vi "Main_without_temperature.vi"() -> ()   [LabVIEW 2023]
uses:
  TEC LabVIEW Control Software v0.14/Source/LV Source/[meerstetter engineering TE Cooling]/TypeDefs/meTEC_ID 2000_Input Selection.ctl
  TEC LabVIEW Control Software v0.14/Source/LV Source/[meerstetter engineering TE Cooling]/TypeDefs/meTEC_ID 50011_Object Target Temperature Source Selection.ctl
  TEC LabVIEW Control Software v0.14/Source/LV Source/[meerstetter engineering TE Cooling]/TypeDefs/meTEC_ID 50000_Live Enable.ctl
  TEC LabVIEW Control Software v0.14/Source/LV Source/[meerstetter engineering TE Cooling]/TypeDefs/meTEC_ID 1200_Temperature is Stable.ctl
  TEC LabVIEW Control Software v0.14/Source/LV Source/[meerstetter engineering TE Cooling]/TypeDefs/meTEC_ID 104_Device Status.ctl
  Application_class/Instruments.ctl
  AD2_MSO_SDK_class/MSOConfig.ctl
  AD2_MSO_SDK_class/AD2TriggerSources.ctl
  AD2_MSO_SDK_class/MSORangeCh.ctl
  Application_class/Control 1.ctl
  Hamamatsu_class/SubRegion.ctl
  Application_class/Application.lvclass
  Dummy_Mtec_class/Dummy_Mtec.lvclass
  C:/GIT/PowerScan/MTEC_Async_class/MTEC_Async.lvclass
  MTEC_Async_class/MTEC_Async.lvclass
  AD2andExtAWG_class/AD2andExtAWG.lvclass
  C:/GIT/PowerScan/InstrumentBase_class/AD2_SDK_class/InstrumentBase.lvclass
  <vilib>/Utility/error.llb/Error Cluster From Error Code.vi
  <vilib>/measure/matone.llb/Extract Single Tone Information 1 Chan.vi
  <vilib>/ErrorRing/Error Ring.xnode
  Hamamatsu_class/Hamamatsu.lvclass
  MTec_class/MTec.lvclass
  InstrumentBase_class/AD2_SDK_class/InstrumentBase.lvclass
  Experiment_class/Experiment.lvclass
  TDMSLogger_PowerScan_class/TDMSLogger_PowerScan.lvclass
  CetoniPump_class/CetoniPump.lvclass
  <vilib>/measure/NI_MAPro.lvlib
  AD2_MSO_SDK_class/AD2_MSO_SDK.lvclass
panel:
  in  "mem size":i32=100
  out "XY Graph":cluster{timestamp[], dbl[]}[](graph)=[{[timestamp(3810714974.4625654 s since 1904-01-01), timestamp(3810714974.6875706 s since 1904-01-01), timestamp(3810714974.9102407 s since 1904-01-01), timestamp(3810714975.132108 s since 1904-01-01), timestamp(3810714975.357173 s since 1904-01-01), timestamp(3810714975.581321 s since 1904-01-01), timestamp(3810714975.80342 s since 1904-01-01), timestamp(3810714976.0264726 s since 1904-01-01), timestamp(3810714976.250123 s since 1904-01-01), timestamp(3810714976.475124 s since 1904-01-01), timestamp(3810714976.6991234 s since 1904-01-01), timestamp(3810714976.9211745 s since 1904-01-01), timestamp(3810714977.1451674 s since 1904-01-01), timestamp(3810714977.368175 s since 1904-01-01), timestamp(3810714977.594176 s since 1904-01-01), timestamp(3810714977.816176 s since 1904-01-01), timestamp(3810714978.0411744 s since 1904-01-01), timestamp(3810714978.263168 s since 1904-01-01), timestamp(3810714978.488388 s since 1904-01-01), timestamp(3810714978.7113824 s since 1904-01-01), timestamp(3810714978.9333825 s since 1904-01-01), timestamp(3810714979.156552 s since 1904-01-01), timestamp(3810714979.380552 s since 1904-01-01), timestamp(3810714979.6040554 s since 1904-01-01), timestamp(3810714979.828112 s since 1904-01-01), timestamp(3810714980.051219 s since 1904-01-01), timestamp(3810714980.275273 s since 1904-01-01), timestamp(3810714980.499636 s since 1904-01-01), timestamp(3810714980.7226286 s since 1904-01-01), timestamp(3810714980.945965 s since 1904-01-01), timestamp(3810714981.170967 s since 1904-01-01), timestamp(3810714981.3933506 s since 1904-01-01), timestamp(3810714981.617357 s since 1904-01-01), timestamp(3810714981.840452 s since 1904-01-01), timestamp(3810714982.0654736 s since 1904-01-01), timestamp(3810714982.2894735 s since 1904-01-01), timestamp(3810714982.510492 s since 1904-01-01), timestamp(3810714982.734492 s since 1904-01-01), timestamp(3810714982.9584928 s since 1904-01-01), timestamp(3810714983.182848 s since 1904-01-01), timestamp(3810714983.4048495 s since 1904-01-01), timestamp(3810714983.6292033 s since 1904-01-01), timestamp(3810714983.8542337 s since 1904-01-01), timestamp(3810714984.077241 s since 1904-01-01), timestamp(3810714984.29924 s since 1904-01-01), timestamp(3810714984.52324 s since 1904-01-01), timestamp(3810714984.7462335 s since 1904-01-01), timestamp(3810714984.9702344 s since 1904-01-01), timestamp(3810714985.195372 s since 1904-01-01), timestamp(3810714985.417372 s since 1904-01-01), timestamp(3810714985.6413646 s since 1904-01-01), timestamp(3810714985.86677 s since 1904-01-01), timestamp(3810714986.0896926 s since 1904-01-01), timestamp(3810714986.311692 s since 1904-01-01), timestamp(3810714986.5356846 s since 1904-01-01), timestamp(3810714986.7598567 s since 1904-01-01), timestamp(3810714986.9828496 s since 1904-01-01), timestamp(3810714987.2071743 s since 1904-01-01), timestamp(3810714987.4291744 s since 1904-01-01), timestamp(3810714987.653329 s since 1904-01-01), timestamp(3810714987.8773217 s since 1904-01-01), timestamp(3810714988.1004457 s since 1904-01-01), timestamp(3810714988.325448 s since 1904-01-01), timestamp(3810714988.547662 s since 1904-01-01), timestamp(3810714988.7716546 s since 1904-01-01), timestamp(3810714988.994662 s since 1904-01-01), timestamp(3810714989.217661 s since 1904-01-01), timestamp(3810714989.443828 s since 1904-01-01), timestamp(3810714989.666828 s since 1904-01-01), timestamp(3810714989.890928 s since 1904-01-01), timestamp(3810714990.11292 s since 1904-01-01), timestamp(3810714990.335927 s since 1904-01-01), timestamp(3810714990.55996 s since 1904-01-01), timestamp(3810714990.7829666 s since 1904-01-01), timestamp(3810714991.006976 s since 1904-01-01), timestamp(3810714991.2310686 s since 1904-01-01), timestamp(3810714991.454176 s since 1904-01-01), timestamp(3810714991.679184 s since 1904-01-01), timestamp(3810714991.903184 s since 1904-01-01), timestamp(3810714992.125177 s since 1904-01-01), timestamp(3810714992.348177 s since 1904-01-01), timestamp(3810714992.572276 s since 1904-01-01), timestamp(3810714992.7962766 s since 1904-01-01), timestamp(3810714993.0195527 s since 1904-01-01), timestamp(3810714993.242547 s since 1904-01-01), timestamp(3810714993.4665465 s since 1904-01-01), timestamp(3810714993.6905394 s since 1904-01-01), timestamp(3810714993.913547 s since 1904-01-01), timestamp(3810714994.1385465 s since 1904-01-01), timestamp(3810714994.3625464 s since 1904-01-01), timestamp(3810714994.585547 s since 1904-01-01), timestamp(3810714994.80954 s since 1904-01-01), timestamp(3810714995.0335464 s since 1904-01-01), timestamp(3810714995.257552 s since 1904-01-01), timestamp(3810714995.4805474 s since 1904-01-01), timestamp(3810714995.7045465 s since 1904-01-01), timestamp(3810714995.925547 s since 1904-01-01), timestamp(3810714996.150547 s since 1904-01-01), timestamp(3810714996.374549 s since 1904-01-01), timestamp(3810714996.596541 s since 1904-01-01)], [22.902175903320312, 22.901992797851562, 22.903213500976562, 22.902908325195312, 22.903305053710938, 22.905197143554688, 22.906875610351562, 22.906539916992188, 22.906539916992188, 22.909378051757812, 22.910781860351562, 22.912826538085938, 22.915451049804688, 22.914047241210938, 22.917343139648438, 22.918472290039062, 22.918655395507812, 22.921981811523438, 22.920059204101562, 22.919723510742188, 22.918167114257812, 22.916549682617188, 22.915725708007812, 22.916458129882812, 22.916946411132812, 22.919662475585938, 22.916976928710938, 22.919906616210938, 22.921005249023438, 22.921249389648438, 22.922714233398438, 22.920883178710938, 22.924118041992188, 22.925735473632812, 22.928085327148438, 22.926986694335938, 22.929306030273438, 22.931716918945312, 22.930801391601562, 22.935470581054688, 22.936508178710938, 22.937179565429688, 22.939346313476562, 22.941116333007812, 22.940444946289062, 22.944534301757812, 22.943649291992188, 22.945999145507812, 22.944869995117188, 22.945846557617188, 22.945571899414062, 22.947494506835938, 22.948379516601562, 22.951004028320312, 22.948989868164062, 22.950271606445312, 22.950210571289062, 22.952072143554688, 22.951004028320312, 22.953475952148438, 22.954299926757812, 22.954116821289062, 22.953506469726562, 22.953598022460938, 22.954208374023438, 22.951828002929688, 22.953872680664062, 22.953018188476562, 22.953842163085938, 22.952865600585938, 22.955795288085938, 22.954513549804688, 22.955978393554688, 22.957351684570312, 22.954727172851562, 22.955886840820312, 22.955001831054688, 22.955825805664062, 22.954360961914062, 22.955032348632812, 22.957229614257812, 22.955490112304688, 22.958755493164062, 22.959518432617188, 22.959548950195312, 22.956710815429688, 22.959915161132812, 22.959487915039062, 22.959426879882812, 22.960617065429688, 22.960525512695312, 22.959243774414062, 22.960983276367188, 22.960647583007812, 22.962112426757812, 22.964004516601562, 22.964279174804688, 22.965377807617188, 22.964614868164062, 22.965621948242188]}, {[timestamp(3810714974.4625654 s since 1904-01-01), timestamp(3810714974.6875706 s since 1904-01-01), timestamp(3810714974.9102407 s since 1904-01-01), timestamp(3810714975.132108 s since 1904-01-01), timestamp(3810714975.357173 s since 1904-01-01), timestamp(3810714975.581321 s since 1904-01-01), timestamp(3810714975.80342 s since 1904-01-01), timestamp(3810714976.0264726 s since 1904-01-01), timestamp(3810714976.250123 s since 1904-01-01), timestamp(3810714976.475124 s since 1904-01-01), timestamp(3810714976.6991234 s since 1904-01-01), timestamp(3810714976.9211745 s since 1904-01-01), timestamp(3810714977.1451674 s since 1904-01-01), timestamp(3810714977.368175 s since 1904-01-01), timestamp(3810714977.594176 s since 1904-01-01), timestamp(3810714977.816176 s since 1904-01-01), timestamp(3810714978.0411744 s since 1904-01-01), timestamp(3810714978.263168 s since 1904-01-01), timestamp(3810714978.488388 s since 1904-01-01), timestamp(3810714978.7113824 s since 1904-01-01), timestamp(3810714978.9333825 s since 1904-01-01), timestamp(3810714979.156552 s since 1904-01-01), timestamp(3810714979.380552 s since 1904-01-01), timestamp(3810714979.6040554 s since 1904-01-01), timestamp(3810714979.828112 s since 1904-01-01), timestamp(3810714980.051219 s since 1904-01-01), timestamp(3810714980.275273 s since 1904-01-01), timestamp(3810714980.499636 s since 1904-01-01), timestamp(3810714980.7226286 s since 1904-01-01), timestamp(3810714980.945965 s since 1904-01-01), timestamp(3810714981.170967 s since 1904-01-01), timestamp(3810714981.3933506 s since 1904-01-01), timestamp(3810714981.617357 s since 1904-01-01), timestamp(3810714981.840452 s since 1904-01-01), timestamp(3810714982.0654736 s since 1904-01-01), timestamp(3810714982.2894735 s since 1904-01-01), timestamp(3810714982.510492 s since 1904-01-01), timestamp(3810714982.734492 s since 1904-01-01), timestamp(3810714982.9584928 s since 1904-01-01), timestamp(3810714983.182848 s since 1904-01-01), timestamp(3810714983.4048495 s since 1904-01-01), timestamp(3810714983.6292033 s since 1904-01-01), timestamp(3810714983.8542337 s since 1904-01-01), timestamp(3810714984.077241 s since 1904-01-01), timestamp(3810714984.29924 s since 1904-01-01), timestamp(3810714984.52324 s since 1904-01-01), timestamp(3810714984.7462335 s since 1904-01-01), timestamp(3810714984.9702344 s since 1904-01-01), timestamp(3810714985.195372 s since 1904-01-01), timestamp(3810714985.417372 s since 1904-01-01), timestamp(3810714985.6413646 s since 1904-01-01), timestamp(3810714985.86677 s since 1904-01-01), timestamp(3810714986.0896926 s since 1904-01-01), timestamp(3810714986.311692 s since 1904-01-01), timestamp(3810714986.5356846 s since 1904-01-01), timestamp(3810714986.7598567 s since 1904-01-01), timestamp(3810714986.9828496 s since 1904-01-01), timestamp(3810714987.2071743 s since 1904-01-01), timestamp(3810714987.4291744 s since 1904-01-01), timestamp(3810714987.653329 s since 1904-01-01), timestamp(3810714987.8773217 s since 1904-01-01), timestamp(3810714988.1004457 s since 1904-01-01), timestamp(3810714988.325448 s since 1904-01-01), timestamp(3810714988.547662 s since 1904-01-01), timestamp(3810714988.7716546 s since 1904-01-01), timestamp(3810714988.994662 s since 1904-01-01), timestamp(3810714989.217661 s since 1904-01-01), timestamp(3810714989.443828 s since 1904-01-01), timestamp(3810714989.666828 s since 1904-01-01), timestamp(3810714989.890928 s since 1904-01-01), timestamp(3810714990.11292 s since 1904-01-01), timestamp(3810714990.335927 s since 1904-01-01), timestamp(3810714990.55996 s since 1904-01-01), timestamp(3810714990.7829666 s since 1904-01-01), timestamp(3810714991.006976 s since 1904-01-01), timestamp(3810714991.2310686 s since 1904-01-01), timestamp(3810714991.454176 s since 1904-01-01), timestamp(3810714991.679184 s since 1904-01-01), timestamp(3810714991.903184 s since 1904-01-01), timestamp(3810714992.125177 s since 1904-01-01), timestamp(3810714992.348177 s since 1904-01-01), timestamp(3810714992.572276 s since 1904-01-01), timestamp(3810714992.7962766 s since 1904-01-01), timestamp(3810714993.0195527 s since 1904-01-01), timestamp(3810714993.242547 s since 1904-01-01), timestamp(3810714993.4665465 s since 1904-01-01), timestamp(3810714993.6905394 s since 1904-01-01), timestamp(3810714993.913547 s since 1904-01-01), timestamp(3810714994.1385465 s since 1904-01-01), timestamp(3810714994.3625464 s since 1904-01-01), timestamp(3810714994.585547 s since 1904-01-01), timestamp(3810714994.80954 s since 1904-01-01), timestamp(3810714995.0335464 s since 1904-01-01), timestamp(3810714995.257552 s since 1904-01-01), timestamp(3810714995.4805474 s since 1904-01-01), timestamp(3810714995.7045465 s since 1904-01-01), timestamp(3810714995.925547 s since 1904-01-01), timestamp(3810714996.150547 s since 1904-01-01), timestamp(3810714996.374549 s since 1904-01-01), timestamp(3810714996.596541 s since 1904-01-01)], [23.093063354492188, 23.094924926757812, 23.094497680664062, 23.097518920898438, 23.095504760742188, 23.094528198242188, 23.098098754882812, 23.099533081054688, 23.102035522460938, 23.100082397460938, 23.105026245117188, 23.107894897460938, 23.107254028320312, 23.108169555664062, 23.112472534179688, 23.110580444335938, 23.116165161132812, 23.113418579101562, 23.113418579101562, 23.112075805664062, 23.110916137695312, 23.108871459960938, 23.107559204101562, 23.110641479492188, 23.111648559570312, 23.111618041992188, 23.113174438476562, 23.115737915039062, 23.115188598632812, 23.116897583007812, 23.113906860351562, 23.116683959960938, 23.119857788085938, 23.119705200195312, 23.120559692382812, 23.123886108398438, 23.123031616210938, 23.122512817382812, 23.124221801757812, 23.128158569335938, 23.127243041992188, 23.129959106445312, 23.131637573242188, 23.131820678710938, 23.133285522460938, 23.136337280273438, 23.136276245117188, 23.136917114257812, 23.138320922851562, 23.137313842773438, 23.141921997070312, 23.142196655273438, 23.142440795898438, 23.143112182617188, 23.145858764648438, 23.144485473632812, 23.147598266601562, 23.147171020507812, 23.149276733398438, 23.149337768554688, 23.149276733398438, 23.152023315429688, 23.155258178710938, 23.155410766601562, 23.153366088867188, 23.155471801757812, 23.154800415039062, 23.155899047851562, 23.157669067382812, 23.159255981445312, 23.157211303710938, 23.157821655273438, 23.160781860351562, 23.162673950195312, 23.161300659179688, 23.164657592773438, 23.164108276367188, 23.163711547851562, 23.162490844726562, 23.165390014648438, 23.165481567382812, 23.165939331054688, 23.165573120117188, 23.169692993164062, 23.168869018554688, 23.167984008789062, 23.168258666992188, 23.168411254882812, 23.168258666992188, 23.168899536132812, 23.170425415039062, 23.170089721679688, 23.171829223632812, 23.173904418945312, 23.172744750976562, 23.175460815429688, 23.173141479492188, 23.174606323242188, 23.174728393554688, 23.175674438476562]}, {[timestamp(3810714974.4625654 s since 1904-01-01), timestamp(3810714974.6875706 s since 1904-01-01), timestamp(3810714974.9102407 s since 1904-01-01), timestamp(3810714975.132108 s since 1904-01-01), timestamp(3810714975.357173 s since 1904-01-01), timestamp(3810714975.581321 s since 1904-01-01), timestamp(3810714975.80342 s since 1904-01-01), timestamp(3810714976.0264726 s since 1904-01-01), timestamp(3810714976.250123 s since 1904-01-01), timestamp(3810714976.475124 s since 1904-01-01), timestamp(3810714976.6991234 s since 1904-01-01), timestamp(3810714976.9211745 s since 1904-01-01), timestamp(3810714977.1451674 s since 1904-01-01), timestamp(3810714977.368175 s since 1904-01-01), timestamp(3810714977.594176 s since 1904-01-01), timestamp(3810714977.816176 s since 1904-01-01), timestamp(3810714978.0411744 s since 1904-01-01), timestamp(3810714978.263168 s since 1904-01-01), timestamp(3810714978.488388 s since 1904-01-01), timestamp(3810714978.7113824 s since 1904-01-01), timestamp(3810714978.9333825 s since 1904-01-01), timestamp(3810714979.156552 s since 1904-01-01), timestamp(3810714979.380552 s since 1904-01-01), timestamp(3810714979.6040554 s since 1904-01-01), timestamp(3810714979.828112 s since 1904-01-01), timestamp(3810714980.051219 s since 1904-01-01), timestamp(3810714980.275273 s since 1904-01-01), timestamp(3810714980.499636 s since 1904-01-01), timestamp(3810714980.7226286 s since 1904-01-01), timestamp(3810714980.945965 s since 1904-01-01), timestamp(3810714981.170967 s since 1904-01-01), timestamp(3810714981.3933506 s since 1904-01-01), timestamp(3810714981.617357 s since 1904-01-01), timestamp(3810714981.840452 s since 1904-01-01), timestamp(3810714982.0654736 s since 1904-01-01), timestamp(3810714982.2894735 s since 1904-01-01), timestamp(3810714982.510492 s since 1904-01-01), timestamp(3810714982.734492 s since 1904-01-01), timestamp(3810714982.9584928 s since 1904-01-01), timestamp(3810714983.182848 s since 1904-01-01), timestamp(3810714983.4048495 s since 1904-01-01), timestamp(3810714983.6292033 s since 1904-01-01), timestamp(3810714983.8542337 s since 1904-01-01), timestamp(3810714984.077241 s since 1904-01-01), timestamp(3810714984.29924 s since 1904-01-01), timestamp(3810714984.52324 s since 1904-01-01), timestamp(3810714984.7462335 s since 1904-01-01), timestamp(3810714984.9702344 s since 1904-01-01), timestamp(3810714985.195372 s since 1904-01-01), timestamp(3810714985.417372 s since 1904-01-01), timestamp(3810714985.6413646 s since 1904-01-01), timestamp(3810714985.86677 s since 1904-01-01), timestamp(3810714986.0896926 s since 1904-01-01), timestamp(3810714986.311692 s since 1904-01-01), timestamp(3810714986.5356846 s since 1904-01-01), timestamp(3810714986.7598567 s since 1904-01-01), timestamp(3810714986.9828496 s since 1904-01-01), timestamp(3810714987.2071743 s since 1904-01-01), timestamp(3810714987.4291744 s since 1904-01-01), timestamp(3810714987.653329 s since 1904-01-01), timestamp(3810714987.8773217 s since 1904-01-01), timestamp(3810714988.1004457 s since 1904-01-01), timestamp(3810714988.325448 s since 1904-01-01), timestamp(3810714988.547662 s since 1904-01-01), timestamp(3810714988.7716546 s since 1904-01-01), timestamp(3810714988.994662 s since 1904-01-01), timestamp(3810714989.217661 s since 1904-01-01), timestamp(3810714989.443828 s since 1904-01-01), timestamp(3810714989.666828 s since 1904-01-01), timestamp(3810714989.890928 s since 1904-01-01), timestamp(3810714990.11292 s since 1904-01-01), timestamp(3810714990.335927 s since 1904-01-01), timestamp(3810714990.55996 s since 1904-01-01), timestamp(3810714990.7829666 s since 1904-01-01), timestamp(3810714991.006976 s since 1904-01-01), timestamp(3810714991.2310686 s since 1904-01-01), timestamp(3810714991.454176 s since 1904-01-01), timestamp(3810714991.679184 s since 1904-01-01), timestamp(3810714991.903184 s since 1904-01-01), timestamp(3810714992.125177 s since 1904-01-01), timestamp(3810714992.348177 s since 1904-01-01), timestamp(3810714992.572276 s since 1904-01-01), timestamp(3810714992.7962766 s since 1904-01-01), timestamp(3810714993.0195527 s since 1904-01-01), timestamp(3810714993.242547 s since 1904-01-01), timestamp(3810714993.4665465 s since 1904-01-01), timestamp(3810714993.6905394 s since 1904-01-01), timestamp(3810714993.913547 s since 1904-01-01), timestamp(3810714994.1385465 s since 1904-01-01), timestamp(3810714994.3625464 s since 1904-01-01), timestamp(3810714994.585547 s since 1904-01-01), timestamp(3810714994.80954 s since 1904-01-01), timestamp(3810714995.0335464 s since 1904-01-01), timestamp(3810714995.257552 s since 1904-01-01), timestamp(3810714995.4805474 s since 1904-01-01), timestamp(3810714995.7045465 s since 1904-01-01), timestamp(3810714995.925547 s since 1904-01-01), timestamp(3810714996.150547 s since 1904-01-01), timestamp(3810714996.374549 s since 1904-01-01), timestamp(3810714996.596541 s since 1904-01-01)], [0.0, 0.0, 0.0, 0.0, 0.0, 0.0, 0.0, 0.0, 0.0, 0.0, 0.0, 0.0, 0.0, 0.0, 0.0, 0.0, 0.0, 0.0, 0.0, 0.0, 0.0, 0.0, 0.0, 0.0, 0.0, 0.0, 0.0, 0.0, 0.0, 0.0, 0.0, 0.0, 0.0, 0.0, 0.0, 0.0, 0.0, 0.0, 0.0, 0.0, 0.0, 0.0, 0.0, 0.0, 0.0, 0.0, 0.0, 0.0, 0.0, 0.0, 0.0, 0.0, 0.0, 0.0, 0.0, 0.0, 0.0, 0.0, 0.0, 0.0, 0.0, 0.0, 0.0, 0.0, 0.0, 0.0, 0.0, 0.0, 0.0, 0.0, 0.0, 0.0, 0.0, 0.0, 0.0, 0.0, 0.0, 0.0, 0.0, 0.0, 0.0, 0.0, 0.0, 0.0, 0.0, 0.0, 0.0, 0.0, 0.0, 0.0, 0.0, 0.0, 0.0, 0.0, 0.0, 0.0, 0.0, 0.0, 0.0, 0.0]}]
  in  "Chart Length":enum16{"60 s", "10 minutes", "1 h"}(ring)=enum."10 minutes"
  out "Waveform Chart":waveform(dbl)[](graph)=[{"t0"=timestamp(3810714996.596541 s since 1904-01-01), "dt"=1.0, "Y"=[22.965621948242188]}, {"t0"=timestamp(3810714996.596541 s since 1904-01-01), "dt"=1.0, "Y"=[23.175674438476562]}]
  in  "Read MSO":bool
  out "error out":errorcluster
  out "Status":string="Exiting.."
  in  "AutoScaleCh1":bool=TRUE caption="AutoScale timebase to ChA"
  out "V/Hz/Deg":dbl[](array[numeric])=[256495.2123849432, 0.012104949851784449, 127.31074154871095, 4268838.632377055, 0.0003381910830981614, 134.9693104826537]
  out "Data":string[](array[string])=["Ch1Freq", "Ch1Amp", "Ch1Phase", "Ch2Freq", "Ch2Amp", "Ch2Phase"]
  out "MSO Data WaveForms 2":waveform(dbl)[](graph)=[{"t0"=timestamp(0 s since 1904-01-01), "dt"=1e-08, "Y"=array[8192 elements]}, {"t0"=timestamp(0 s since 1904-01-01), "dt"=1e-08, "Y"=array[8192 elements]}]
  in  "ABORT":bool
  in  "Tab Control":T1(tab)=enum."Cetoni"
  in  "Use Cetoni?":bool=TRUE
  in  "Use Hamamatsu":bool=TRUE
  in  "Use MeTEC?":bool=TRUE
  in  "AWG VISA resource name":refnum<visa-resource-name>="USB0::0x0699::0x0347::C037907::INSTR"
  in  "System Configuration":T2
  in  "Initialize System":bool
  in  "Use Instruments?":bool=TRUE
  in  "Device Configuration Path":string="C:\\Users\\Public\\Documents\\QmixElements\\Projects\\default_project\\Configurations\\double"
  in  "Turn Off WFG During Refill":bool
  in  "index":i32
  in  "refill below level(uL)":dbl=1000.0
  in  "Refill":bool
  in  "Conditional Refill":bool
  in  "Empty":bool
  in  "Stop pumps":bool
  in  "SyringeSettings":T3={"Maximum Piston Stroke (mm)"=66.0, "Inner Diameter (mm)"=14.5}
  in  "Configure Syringe":bool
  in  "ValveControl":cluster{"index":i32, "Valve Position":bool}
  in  "Go to Level":bool
  in  "GoToLevelSettings":T4={"index"=0, "Level(uL)"=0.0, "Flow"=250.0}
  in  "Monitor Pump":bool
  out "Array":T5(array[cluster])=[{"Pump Name"="neMESYS_Low_Pressure_1_Pump", "Actual Flow Rate"=249.9994261659258, "Fill Level"=9609.141943854513, "Is pumping"=TRUE}, {"Pump Name"="neMESYS_Low_Pressure_2_Pump", "Actual Flow Rate"=0.0, "Fill Level"=0.0, "Is pumping"=FALSE}]
  in  "ReferenceMove":bool
  in  "refill and \nempty rate(uL/min)":dbl=12000.0
  in  "Wait After Conditional Refill (s)":dbl=50.0
  out "Cluster":T8={"meTEC_CH2_Temperature Stability"=0, "meTEC_CH2_Act. Output Current [A]"=0.009997940622270107, "meTEC_CH2_Act. Output Voltage [V]"=0.004072710871696472, "meTEC_CH2_Object Temperature [°C]"=23.175674438476562, "meTEC_CH2_Sink Temperature [°C]"=25.0, "meTEC_CH1_Error Parameter"=0, "meTEC_CH1_Error Instance"=0, "meTEC_CH1_Error No."=0, "meTEC_CH1_Device Status"=1, "meTEC_CH1_Temperature Stability"=0, "meTEC_CH1_Act. Output Current [A]"=0.010120010934770107, "meTEC_CH1_Act. Output Voltage [V]"=0.009891997091472149, "meTEC_CH1_Object Temperature [°C]"=22.965621948242188, "meTEC_CH1_Sink Temperature [°C]"=25.0} {"meTEC_CH1_Sink Temperature [°C]" format="%.3f"; "meTEC_CH1_Object Temperature [°C]" format="%.3f"; "meTEC_CH1_Act. Output Voltage [V]" format="%.3f"; "meTEC_CH1_Act. Output Current [A]" format="%.3f"; "meTEC_CH1_Temperature Stability" items=["Temperature regulation is not active", "Is not stable", "Is stable"]; "meTEC_CH1_Device Status" items=["Initializing", "Ready", "Run", "Error", "Bootloader", "Reset in Progress"]; "meTEC_CH2_Sink Temperature [°C]" format="%.3f"; "meTEC_CH2_Object Temperature [°C]" format="%.3f"; "meTEC_CH2_Act. Output Voltage [V]" format="%.3f"; "meTEC_CH2_Act. Output Current [A]" format="%.3f"; "meTEC_CH2_Temperature Stability" items=["Temperature regulation is not active", "Is not stable", "Is stable"]}
  in  "Config Data":T12={"meTEC_CH1_Input Selection (ID 2000)"=2, "meTEC_CH2_Input Selection (ID 2000)"=2, "meTEC_CH1_Object Target Temp. Source Selection (ID 50011)"=0, "meTEC_CH2_Object Target Temp. Source Selection (ID 50011)"=0, "meTEC_CH1_Live Enable (ID 50000)"=0, "meTEC_CH2_Live Enable (ID 50000)"=0, "meTEC_CH1_Object Target Temperature (ID 3000 / 50012) [°C]"=23.0, "meTEC_CH2_Object Target Temperature (ID 3000 / 50012) [°C]"=23.0, "meTEC_CH1_Live Set Current (ID 50001) [A]"=0.0, "meTEC_CH2_Live Set Current (ID 50001) [A]"=0.0, "meTEC_CH1_Live Set Voltage (ID 50002) [V]"=0.0, "meTEC_CH2_Live Set Voltage (ID 50002) [V]"=0.0} {"meTEC_CH2_Live Set Voltage (ID 50002) [V]" format="%#.3f"; "meTEC_CH1_Live Set Voltage (ID 50002) [V]" format="%#.3f"; "meTEC_CH2_Live Set Current (ID 50001) [A]" format="%#.3f"; "meTEC_CH1_Live Set Current (ID 50001) [A]" format="%#.3f"; "meTEC_CH2_Object Target Temperature (ID 3000 / 50012) [°C]" format="%#.3f"; "meTEC_CH1_Object Target Temperature (ID 3000 / 50012) [°C]" format="%#.3f"; "meTEC_CH2_Live Enable (ID 50000)" items=["Disabled (Reset State)", "Enabled"]; "meTEC_CH1_Live Enable (ID 50000)" items=["Disabled (Reset State)", "Enabled"]; "meTEC_CH2_Object Target Temp. Source Selection (ID 50011)" items=["Parameter ID 3000 (Reset State)", "Parameter ID 50012"]; "meTEC_CH1_Object Target Temp. Source Selection (ID 50011)" items=["Parameter ID 3000 (Reset State)", "Parameter ID 50012"]; "meTEC_CH2_Input Selection (ID 2000)" items=["Static Current / Voltage", "Live Current / Voltage", "Temperature Controller"]; "meTEC_CH1_Input Selection (ID 2000)" items=["Static Current / Voltage", "Live Current / Voltage", "Temperature Controller"]}
  in  "Configure TEC":bool
  in  "Monitor":bool=TRUE
  in  "ResetMtec":bool
  in  "Metec Flush Memory":bool
  in  "OutputEnable":T13
  in  "Config WFG":bool
  in  "Freq Ch1&2":T14
  in  "Configdatastd":T15={"ConfigDataCh1"={"Frequency Hz (1000 Hz)"=1000.0, "Waveform Function (0: Sine)"=0, "Amplitude (1 Vpp)"=1.0, "DC Offset (0.00 V)"=0.0, "Phase Level (-1)"=0.0, "Phase Unit (0: Radian)"=0}, "ConfigDataCh2"={"Frequency Hz (1000 Hz)"=1000.0, "Waveform Function (0: Sine)"=0, "Amplitude (1 Vpp)"=1.0, "DC Offset (0.00 V)"=0.0, "Phase Level (-1)"=0.0, "Phase Unit (0: Radian)"=0}} {"ConfigDataCh1"."Frequency Hz (1000 Hz)" min=0.0 max=100000000.0}
  in  "CurrentProbeScaling(V/A)":dbl=5.0
  in  "PwrScanSettings":T16={"FreqStart(Hz)"=1800000.0, "Increment(Hz)"=1000.0, "Steps"=100}
  out "Power Graph":T17=[{"PwrFreq"=[1800000.0, 1801000.0, 1802000.0, 1803000.0, 1804000.0, 1805000.0, 1806000.0, 1807000.0, 1808000.0, 1809000.0, 1810000.0, 1811000.0, 1812000.0, 1813000.0, 1814000.0, 1815000.0, 1816000.0, 1817000.0, 1818000.0, 1819000.0, 1820000.0, 1821000.0, 1822000.0, 1823000.0, 1824000.0, 1825000.0, 1826000.0, 1827000.0, 1828000.0, 1829000.0, 1830000.0, 1831000.0, 1832000.0, 1833000.0, 1834000.0, 1835000.0, 1836000.0, 1837000.0, 1838000.0, 1839000.0, 1840000.0, 1841000.0, 1842000.0, 1843000.0, 1844000.0, 1845000.0, 1846000.0, 1847000.0, 1848000.0, 1849000.0, 1850000.0, 1851000.0, 1852000.0, 1853000.0, 1854000.0, 1855000.0, 1856000.0, 1857000.0, 1858000.0, 1859000.0, 1860000.0, 1861000.0, 1862000.0, 1863000.0, 1864000.0, 1865000.0, 1866000.0, 1867000.0, 1868000.0, 1869000.0, 1870000.0, 1871000.0, 1872000.0, 1873000.0, 1874000.0, 1875000.0, 1876000.0, 1877000.0, 1878000.0, 1879000.0, 1880000.0, 1881000.0, 1882000.0, 1883000.0, 1884000.0, 1885000.0, 1886000.0, 1887000.0, 1888000.0, 1889000.0, 1890000.0, 1891000.0, 1892000.0, 1893000.0, 1894000.0, 1895000.0, 1896000.0, 1897000.0, 1898000.0, 1899000.0], "PwrMeasured"=[0.03743018699905172, 0.03868842711054406, 0.039939450983681936, 0.041186940846945984, 0.042492363236693975, 0.04404846555067622, 0.04602835102242353, 0.04843888820937301, 0.05119026075250401, 0.054137745072059686, 0.05681989848669318, 0.05866977349663312, 0.05974650294953525, 0.06005376515825572, 0.05994285605916934, 0.05965859181003201, 0.05940789816848652, 0.05911436810870655, 0.05887115083576992, 0.058285278937152116, 0.05733209401753114, 0.05612065814579392, 0.05491201122450486, 0.054246204884069796, 0.05413387963390649, 0.0544784492868222, 0.055223443274043806, 0.05584761484864832, 0.05593777472478643, 0.055604310692913786, 0.05518644597062401, 0.054618464862787694, 0.054214223715299915, 0.05394256784700533, 0.0538322569007853, 0.05378224385812821, 0.053684397213232725, 0.053570515853526054, 0.05367988225271155, 0.05367731285637497, 0.05328103475935342, 0.05261733484260826, 0.05172095371283941, 0.050922021343682664, 0.05021598202266246, 0.049693559571941236, 0.04964157824916153, 0.049770317527984026, 0.04982229343352004, 0.0491940448801376, 0.048088239496034246, 0.0465169483544214, 0.0449815088404273, 0.04339710247015175, 0.04200318845517933, 0.04079371088999795, 0.03986802195324547, 0.038792483453571246, 0.03777766173772913, 0.03677527534117768, 0.0359760414327305, 0.03518671210489007, 0.03475002270949958, 0.03471532342952112, 0.03517735874853088, 0.03613562839997322, 0.0377065106935801, 0.0398207089338458, 0.04192610453201364, 0.04433368155489899, 0.04724045693183674, 0.05041187326865423, 0.05357414254285915, 0.056935687754456586, 0.06034831631771629, 0.06370638524387114, 0.06689701401467622, 0.06907501466358135, 0.07011171729016413, 0.06928919978057443, 0.06697831206028507, 0.06356111518422408, 0.059707919276213384, 0.055820271940164715, 0.05201579594450088, 0.048220123240964884, 0.044549547433591366, 0.04117661978432694, 0.038128405762736364, 0.03561051707739825, 0.03331342696116638, 0.03141526136270806, 0.029497507637866037, 0.02786984120696333, 0.0266553633197663, 0.025619681037449903, 0.024768741920820493, 0.024028995090048973, 0.023324807778494015, 0.022671870223729386]}, {"PwrFreq"=[], "PwrMeasured"=[]}, {"PwrFreq"=[], "PwrMeasured"=[]}]
  in  "AdjustPower":bool
  in  "DesiredPower(W)":dbl=0.001 min=0.001
  out "min Power":dbl=0.022671870223729386
  out "max Power":dbl=0.07011171729016413
  out "Measured Power":dbl=0.014358194668451557
  in  "MeasurePower":bool
  out "AmplitudeOk":bool=TRUE
  in  "Run Power Scan":bool
  out "phase (deg)":dbl=82.9743375382008
  out "impedance (ohm)":dbl=0.07240014859741192
  in  "Config":T18={"Timing"={"Enable"=TRUE, "Samples In"=8000.0, "Sample Rate"=100000000.0, "Mode"=enum."Single Sample"}, "Trigger"={"Hysteresis"=0.0, "Trigger Level"=0.0, "Trigger Condition"=0, "Trigger Type"=0, "Trigger Channel"=0, "secTimeout"=0.5, "TrigrSrc"=enum."trigsrcDetectorAnalogIn"}, "Range Ch1"={"idxChannel"=0, "voltOffset"=0.0, "VoltsRange"=50}, "Range Ch 2"={"idxChannel"=1, "voltOffset"=0.0, "VoltsRange"=5}} {"Range Ch 2"."VoltsRange" items=["High 50V"=50, "Low5V"=5]; "Range Ch1"."VoltsRange" items=["High 50V"=50, "Low5V"=5]; "Trigger"."Trigger Channel" items=["Channel 1"=0, "Channel 2"=1, "Both"=-1]; "Trigger"."Trigger Type" items=["Edge", "Pulse", "Transition"]; "Trigger"."Trigger Condition" items=["Rising", "Falling"]}
  in  "Configure MSO":bool
  in  "AutoRange MSO (Volt)":bool
  in  "Center ROI":bool=TRUE
  in  "Image":bool
  in  "Image Continous":bool
  in  "ExposureTime(ms)":dbl=5.0
  in  "ROI":T21={"Horizontal Offset"=0, "Vertical Offset"=652, "Horizontal Size"=2304, "Vertical Size"=1000} {"Vertical Size" min=4 max=1652 step=4; "Horizontal Size" min=4 max=2304 step=4; "Vertical Offset" min=0 max=1304 step=4; "Horizontal Offset" min=0 max=0 step=4}
  in  "Configure":bool
  in  "Fill List":bool
  in  "Number of Frequencies":dbl=101.0
  in  "Freq Increment":dbl=1000.0
  in  "Freq Start":dbl=1800000.0
  in  "Start Experiment":bool
  in  "Number of Images (#)":i32=10
  in  "wait time(s)":dbl
  in  "List of Powers to run(W)":dbl[](array[numeric])=[0.01, 0.02] min=0.001
  in  "List of Frequencies (Hz)":dbl[](array[numeric])=[1800000.0, 1801000.0, 1802000.0, 1803000.0, 1804000.0, 1805000.0, 1806000.0, 1807000.0, 1808000.0, 1809000.0, 1810000.0, 1811000.0, 1812000.0, 1813000.0, 1814000.0, 1815000.0, 1816000.0, 1817000.0, 1818000.0, 1819000.0, 1820000.0, 1821000.0, 1822000.0, 1823000.0, 1824000.0, 1825000.0, 1826000.0, 1827000.0, 1828000.0, 1829000.0, 1830000.0, 1831000.0, 1832000.0, 1833000.0, 1834000.0, 1835000.0, 1836000.0, 1837000.0, 1838000.0, 1839000.0, 1840000.0, 1841000.0, 1842000.0, 1843000.0, 1844000.0, 1845000.0, 1846000.0, 1847000.0, 1848000.0, 1849000.0, 1850000.0, 1851000.0, 1852000.0, 1853000.0, 1854000.0, 1855000.0, 1856000.0, 1857000.0, 1858000.0, 1859000.0, 1860000.0, 1861000.0, 1862000.0, 1863000.0, 1864000.0, 1865000.0, 1866000.0, 1867000.0, 1868000.0, 1869000.0, 1870000.0, 1871000.0, 1872000.0, 1873000.0, 1874000.0, 1875000.0, 1876000.0, 1877000.0, 1878000.0, 1879000.0, 1880000.0, 1881000.0, 1882000.0, 1883000.0, 1884000.0, 1885000.0, 1886000.0, 1887000.0, 1888000.0, 1889000.0, 1890000.0, 1891000.0, 1892000.0, 1893000.0, 1894000.0, 1895000.0, 1896000.0, 1897000.0, 1898000.0, 1899000.0, 1900000.0] min=0.001
  out "Progress (100%)":dbl=100.0
  in  "List of Flow Rates (ul/min)":dbl[](array[numeric])=[250.0]
  out "# elements in queue":i32=3256
  in  "Repeat Adjust Power and Wait N Times (#)":i32=1 min=1
  in  "wait after adjust power (s)":dbl
  in  "wait after changing flow rate(s)":dbl
  in  "AutoRange MSO":bool
  in  "Exit":bool
  # "All Power Levels"
  # "All Frequencies"
  # "All Flow Rates"
  # "Conditional Refill\nSet Flow\nChange Frequency\nEnable Function Generator\nAdjust Power\nWait (Adjust Power)\nWait\nSave Data (N times)\nDisable Function Generator\nWait\nSave Data"
  # "Measured Waveform"
  # "Index of the pump you are controlling"
  # "This one goes to 11!"
  # "Refills if syringe\nis below level"
  # "(sets it back to its previous state after)"
  # "Volt on ch1 and Current Probe ch2"
  # "(also measures impedance)"
  # "All Power Levels"
  # "All Frequencies"
  # "All Flow Rates"
  # "Conditional Refill\nSet Flow\nWait (flow)\nChange Frequency\nEnable Function Generator\nAdjust Power\nWait (Adjust Power)\nWait\nSave Data (N times)\nDisable Function Generator\nWait\nSave Data"
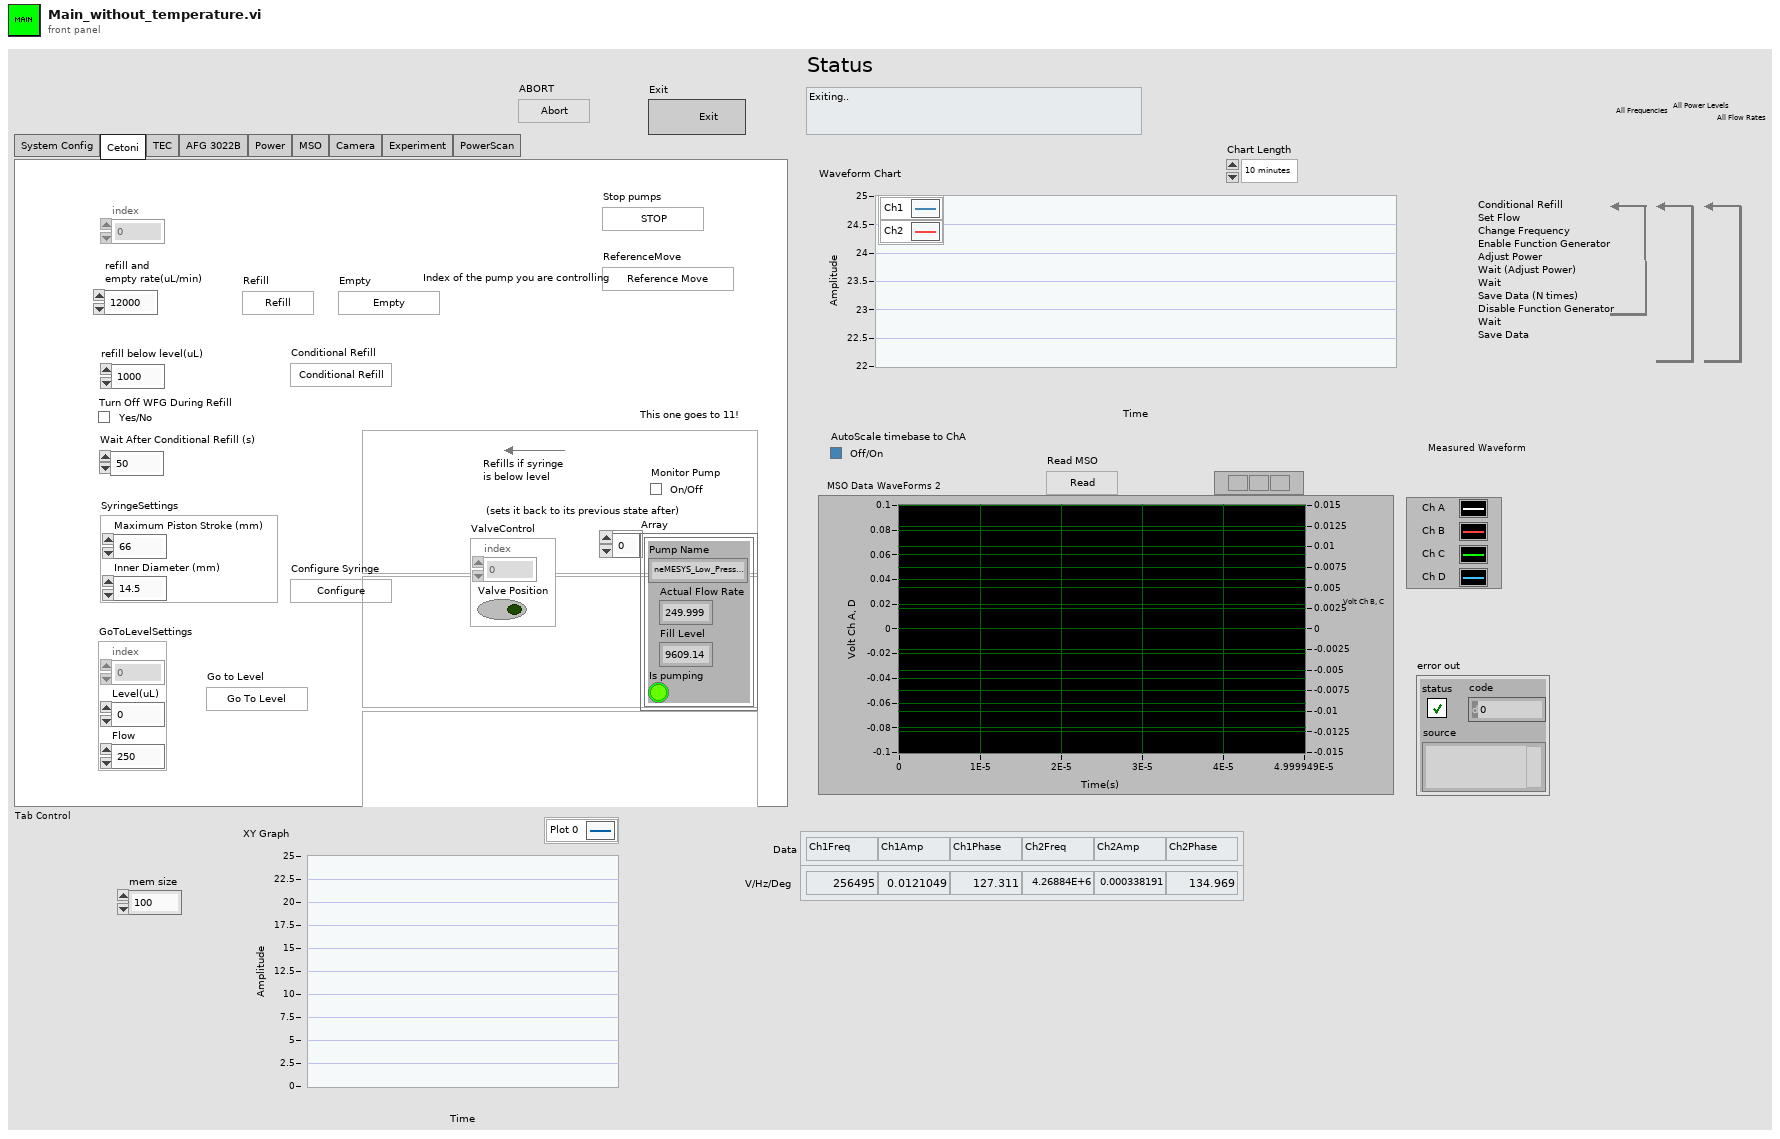
[diagram p1: front panel]
types:
  T1 = enum32{"System Config", "Cetoni", "TEC", "AFG 3022B", "Power", "MSO", "Camera", "Experiment", "PowerScan"}
  T2 = typedef "Application.lvclass/Instruments.ctl" = enum16{"AD2 and AFG3022"}
  T3 = cluster{"Maximum Piston Stroke (mm)":dbl, "Inner Diameter (mm)":dbl}
  T4 = cluster{"index":i32, "Level(uL)":dbl, "Flow":dbl}
  T5 = cluster{"Pump Name":string, "Actual Flow Rate":dbl, "Fill Level":dbl, "Is pumping":bool}[]
  T6 = typedef "meTEC_ID 1200_Temperature is Stable.ctl" = i32
  T7 = typedef "meTEC_ID 104_Device Status.ctl" = i32
  T8 = cluster{"meTEC_CH2_Temperature Stability":T6, "meTEC_CH2_Act. Output Current [A]":dbl, "meTEC_CH2_Act. Output Voltage [V]":dbl, "meTEC_CH2_Object Temperature [°C]":dbl, "meTEC_CH2_Sink Temperature [°C]":dbl, "meTEC_CH1_Error Parameter":i32, "meTEC_CH1_Error Instance":i32, "meTEC_CH1_Error No.":i32, "meTEC_CH1_Device Status":T7, "meTEC_CH1_Temperature Stability":T6, "meTEC_CH1_Act. Output Current [A]":dbl, "meTEC_CH1_Act. Output Voltage [V]":dbl, "meTEC_CH1_Object Temperature [°C]":dbl, "meTEC_CH1_Sink Temperature [°C]":dbl}
  T9 = typedef "meTEC_ID 2000_Input Selection.ctl" = i32
  T10 = typedef "meTEC_ID 50011_Object Target Temperature Source Selection.ctl" = i32
  T11 = typedef "meTEC_ID 50000_Live Enable.ctl" = i32
  T12 = cluster{"meTEC_CH1_Input Selection (ID 2000)":T9, "meTEC_CH2_Input Selection (ID 2000)":T9, "meTEC_CH1_Object Target Temp. Source Selection (ID 50011)":T10, "meTEC_CH2_Object Target Temp. Source Selection (ID 50011)":T10, "meTEC_CH1_Live Enable (ID 50000)":T11, "meTEC_CH2_Live Enable (ID 50000)":T11, "meTEC_CH1_Object Target Temperature (ID 3000 / 50012) [°C]":dbl, "meTEC_CH2_Object Target Temperature (ID 3000 / 50012) [°C]":dbl, "meTEC_CH1_Live Set Current (ID 50001) [A]":dbl, "meTEC_CH2_Live Set Current (ID 50001) [A]":dbl, "meTEC_CH1_Live Set Voltage (ID 50002) [V]":dbl, "meTEC_CH2_Live Set Voltage (ID 50002) [V]":dbl}
  T13 = cluster{"Enable Output WFG Ch1":bool, "Enable Output WFG Ch 2":bool}
  T14 = cluster{"Ch1.Carrier.Frequency (Hz)":dbl, "Ch2.Carrier.Frequency (Hz)":dbl}
  T15 = cluster{"ConfigDataCh1":cluster{"Frequency Hz (1000 Hz)":dbl, "Waveform Function (0: Sine)":u16, "Amplitude (1 Vpp)":dbl, "DC Offset (0.00 V)":dbl, "Phase Level (-1)":dbl, "Phase Unit (0: Radian)":u16}, "ConfigDataCh2":cluster{"Frequency Hz (1000 Hz)":dbl, "Waveform Function (0: Sine)":u16, "Amplitude (1 Vpp)":dbl, "DC Offset (0.00 V)":dbl, "Phase Level (-1)":dbl, "Phase Unit (0: Radian)":u16}}
  T16 = cluster{"FreqStart(Hz)":dbl, "Increment(Hz)":dbl, "Steps":i32}
  T17 = typedef "Control 1.ctl" = cluster{"PwrFreq":dbl[], "PwrMeasured":dbl[]}[]
  T18 = typedef "AD2_MSO_SDK.lvclass/MSOConfig.ctl" = cluster{"Timing":cluster{"Enable":bool, "Samples In":dbl, "Sample Rate":dbl, "Mode":enum16{"Single Sample", "Scanshift", "Multiple Samples", "Scan Screen"}}, "Trigger":cluster{"Hysteresis":dbl, "Trigger Level":dbl, "Trigger Condition":i32, "Trigger Type":i32, "Trigger Channel":i32, "secTimeout":dbl, "TrigrSrc":T19}, "Range Ch1":T20, "Range Ch 2":T20}
  T19 = typedef "AD2_MSO_SDK.lvclass/AD2TriggerSources.ctl" = enum8{"trigrsrcNone", "trigsrcPC", "trigsrcDetectorAnalogIn", "trigsrcDetectorDigitalIn", "trigsrcAnalogIn", "trigsrcDigitalIn", "trigsrcDigitalOut", "trigsrcAnalogOut1", "trigsrcAnalogOut2", "trigsrcAnalogOut3", "trigsrcAnalogOut4", "trigsrcExternal1", "trigsrcExternal2", "trigsrcExternal3", "trigsrcExternal4", ""}
  T20 = typedef "AD2_MSO_SDK.lvclass/MSORangeCh.ctl" = cluster{"idxChannel":i32, "voltOffset":dbl, "VoltsRange":u16}
  T21 = typedef "Hamamatsu.lvclass/SubRegion.ctl" = cluster{"Horizontal Offset":i32, "Vertical Offset":i32, "Horizontal Size":i32, "Vertical Size":i32}
  T22 = cluster{"index":i32, "Level(ml)":dbl, "Flow":dbl}
  T23 = typedef "LVMinMaxIncTypeDef.ctl" = cluster{"Minimum":dbl, "Maximum":dbl, "Increment":dbl}
  T24 = cluster{"H Offset":cluster{"Value":i32, "Limits":T23}, "V Offset":cluster{"Value":i32, "Limits":T23}, "H Size":cluster{"Value":i32, "Limits":T23}, "V Size":cluster{"Value":i32, "Limits":T23}}
  T25 = typedef "Hamamatsu.lvclass/SubRegionLimits.ctl" = cluster{"H Offset":cluster{"Value":i32, "Limits":T23}, "V Offset":cluster{"Value":i32, "Limits":T23}, "H Size":cluster{"Value":i32, "Limits":T23}, "V Size":cluster{"Value":i32, "Limits":T23}}
  T26 = typedef "IMAQ Image.ctl" = refnum<image>
  T27 = cluster{"current time":timestamp, "DataOut":cluster{"meTEC_CH2_Temperature Stability":T6, "meTEC_CH2_Act. Output Current [A]":dbl, "meTEC_CH2_Act. Output Voltage [V]":dbl, "meTEC_CH2_Object Temperature [°C]":dbl, "meTEC_CH2_Sink Temperature [°C]":dbl, "meTEC_CH1_Error Parameter":i32, "meTEC_CH1_Error Instance":i32, "meTEC_CH1_Error No.":i32, "meTEC_CH1_Device Status":T7, "meTEC_CH1_Temperature Stability":T6, "meTEC_CH1_Act. Output Current [A]":dbl, "meTEC_CH1_Act. Output Voltage [V]":dbl, "meTEC_CH1_Object Temperature [°C]":dbl, "meTEC_CH1_Sink Temperature [°C]":dbl}}
  T28 = cluster{"current time":timestamp, "DataOut":cluster{"meTEC_CH2_Temperature Stability":T6, "meTEC_CH2_Act. Output Current [A]":dbl, "meTEC_CH2_Act. Output Voltage [V]":dbl, "meTEC_CH2_Object Temperature [°C]":dbl, "meTEC_CH2_Sink Temperature [°C]":dbl, "meTEC_CH1_Error Parameter":i32, "meTEC_CH1_Error Instance":i32, "meTEC_CH1_Error No.":i32, "meTEC_CH1_Device Status":T7, "meTEC_CH1_Temperature Stability":T6, "meTEC_CH1_Act. Output Current [A]":dbl, "meTEC_CH1_Act. Output Voltage [V]":dbl, "meTEC_CH1_Object Temperature [°C]":dbl, "meTEC_CH1_Sink Temperature [°C]":dbl}}[]
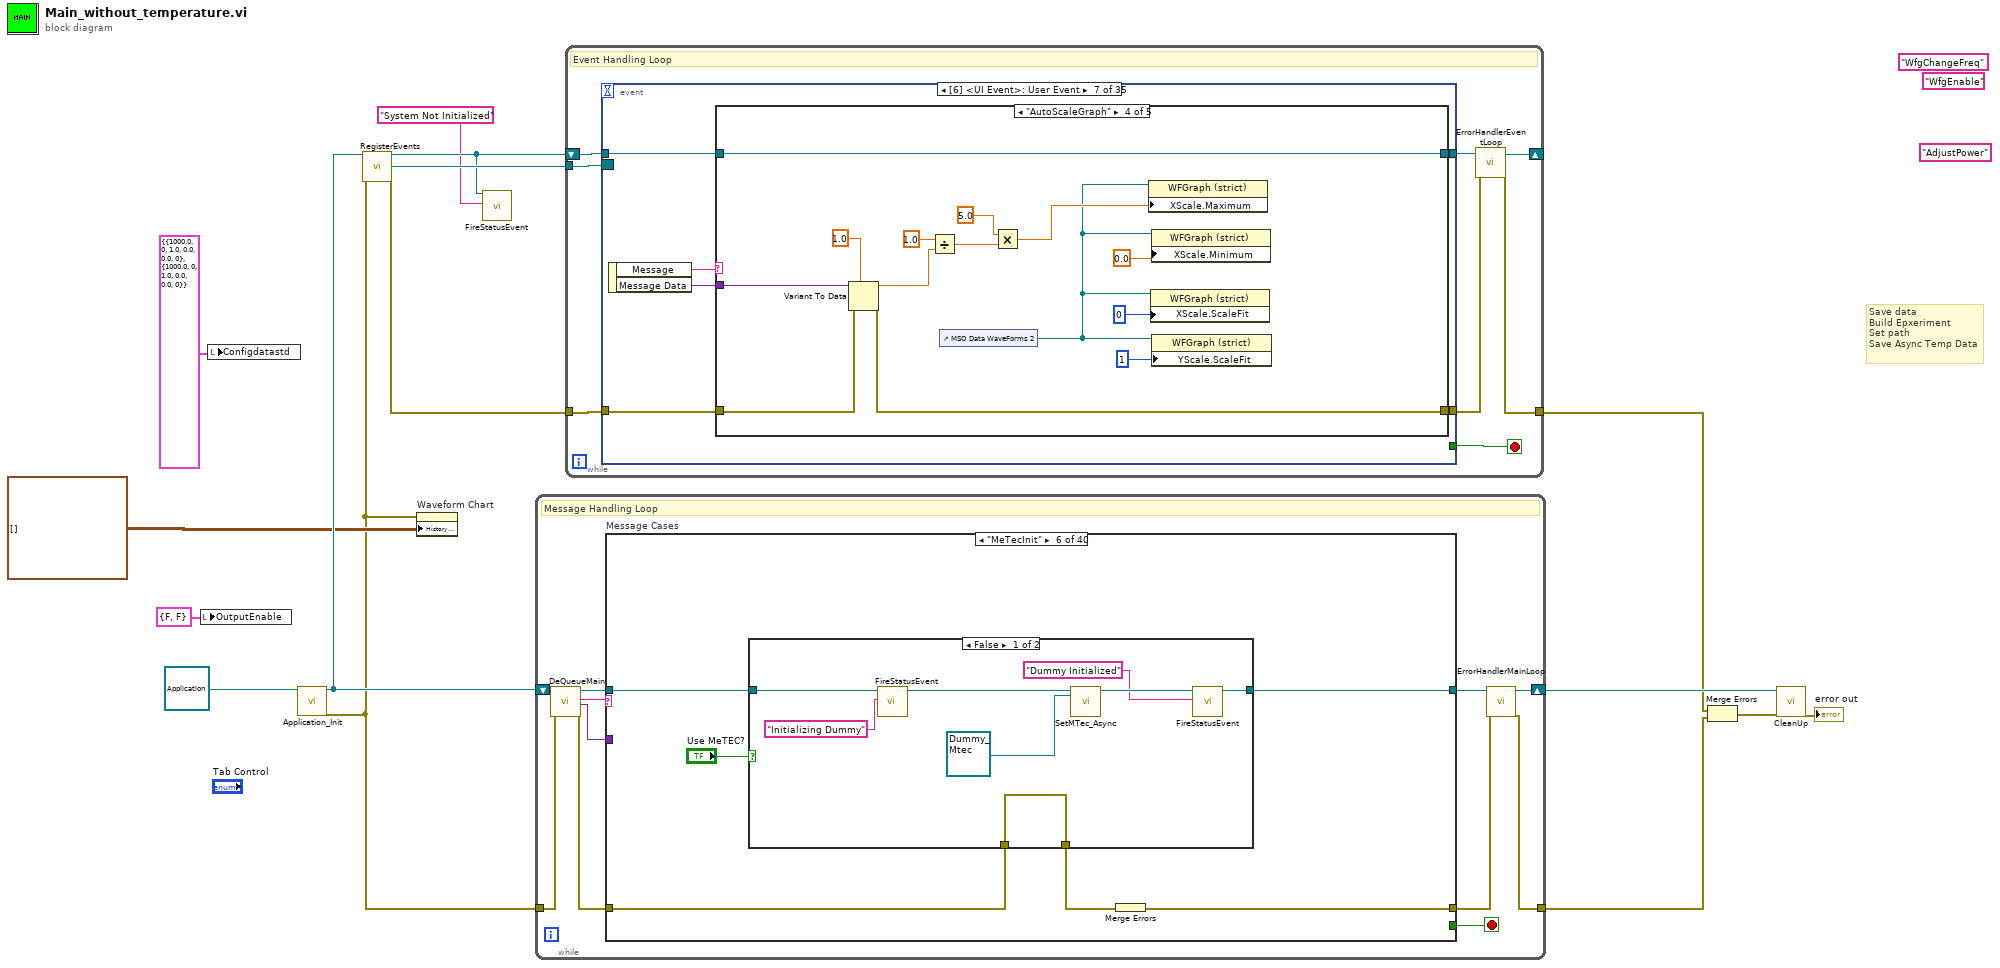
[diagram p0: block diagram]
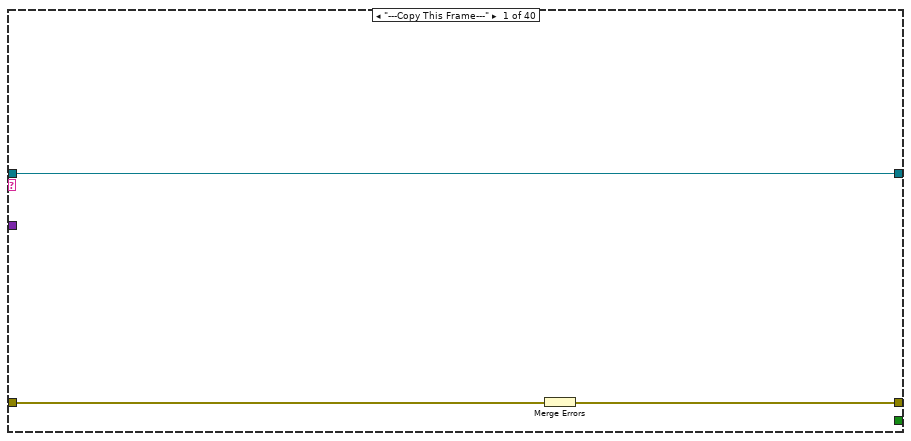
[diagram p2: hidden frame]
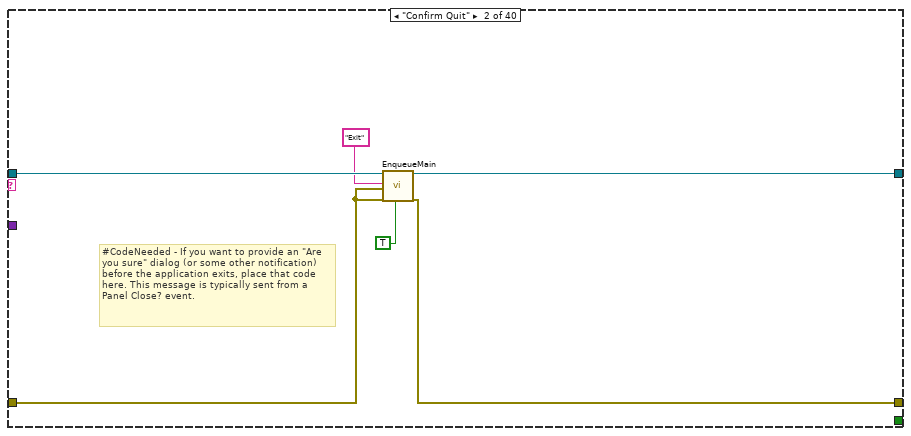
[diagram p3: hidden frame]
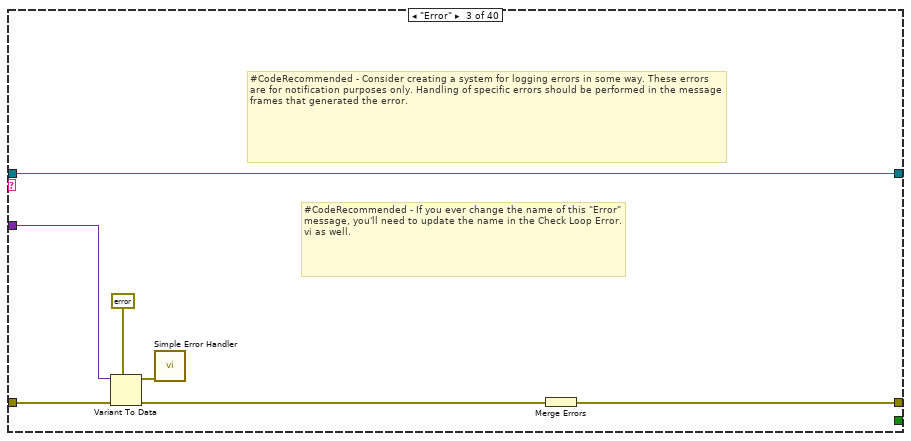
[diagram p4: hidden frame]
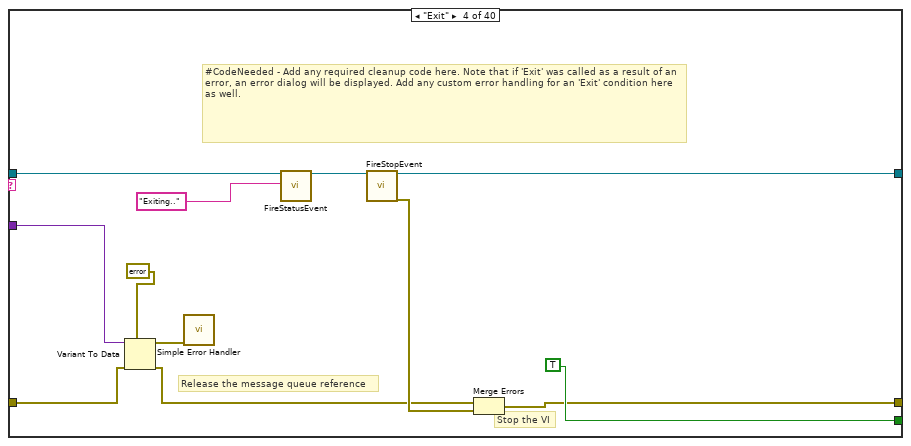
[diagram p5: hidden frame]
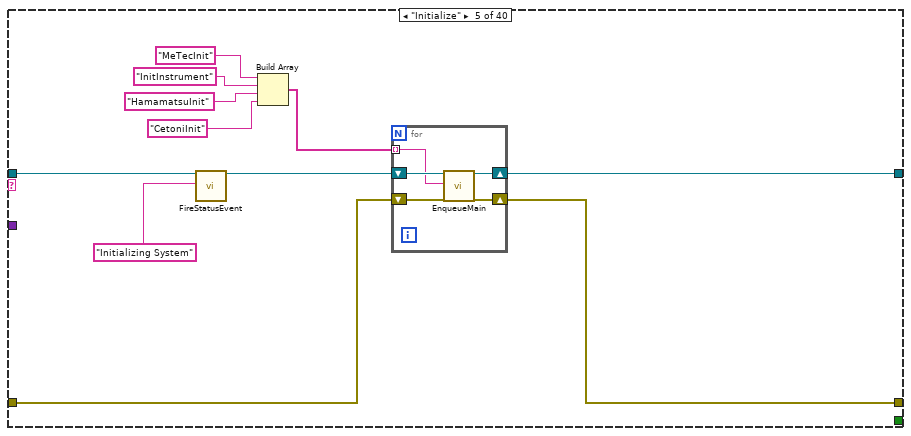
[diagram p6: hidden frame]
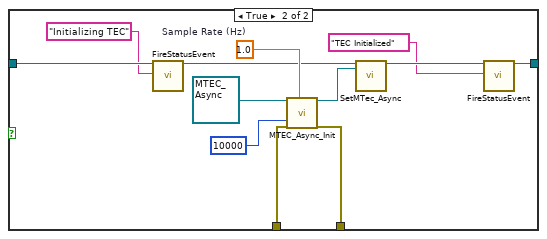
[diagram p7: hidden frame]
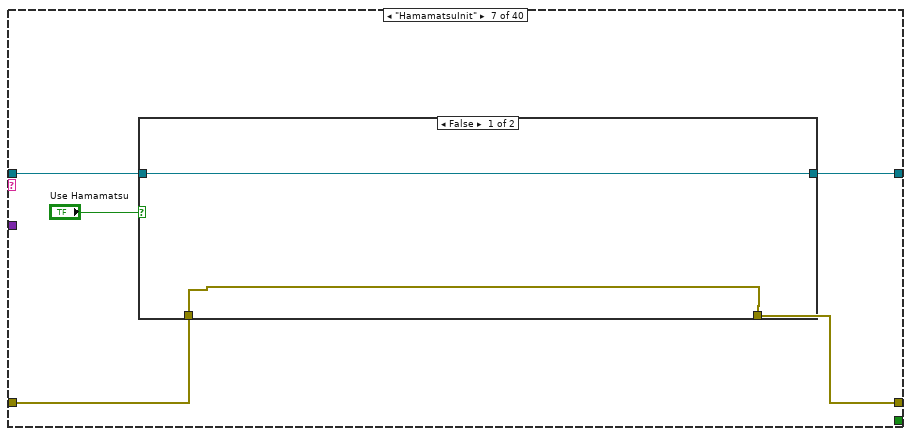
[diagram p8: hidden frame]
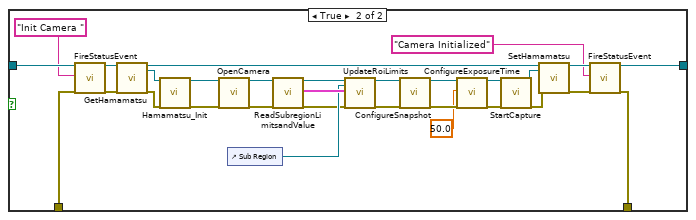
[diagram p9: hidden frame]
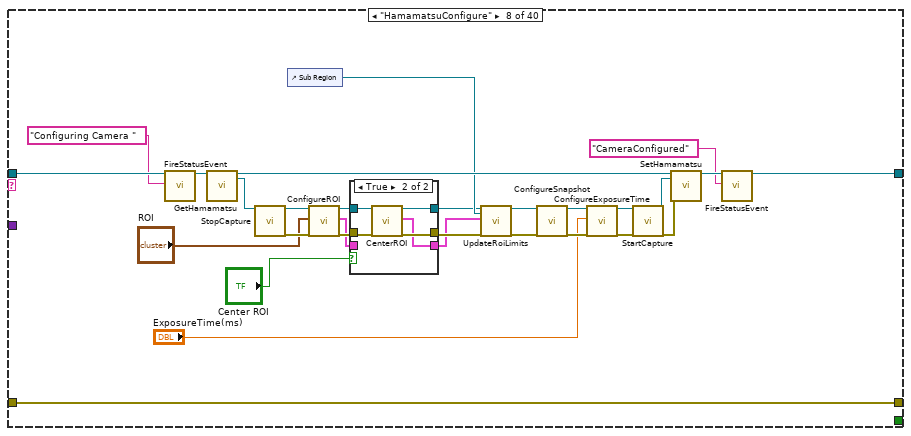
[diagram p10: hidden frame]
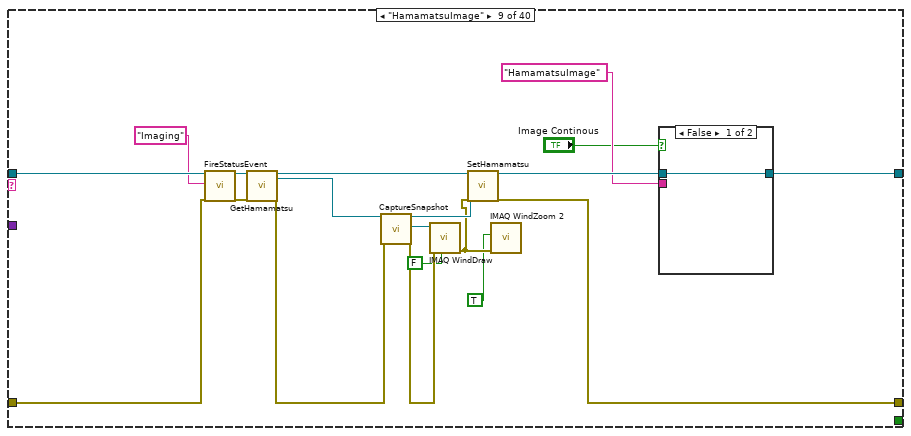
[diagram p12: hidden frame]
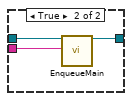
[diagram p13: hidden frame]
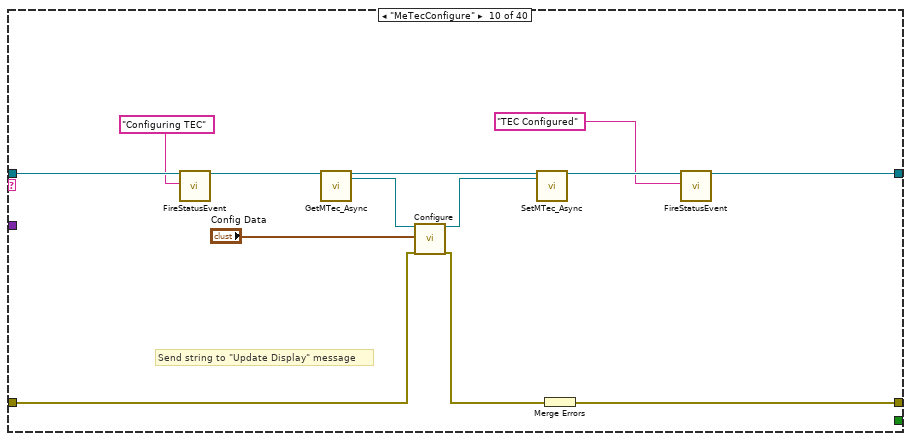
[diagram p14: hidden frame]
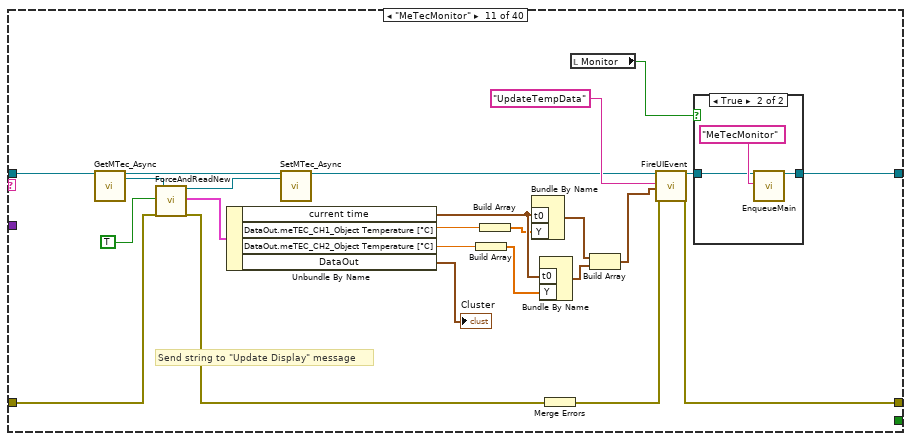
[diagram p15: hidden frame]
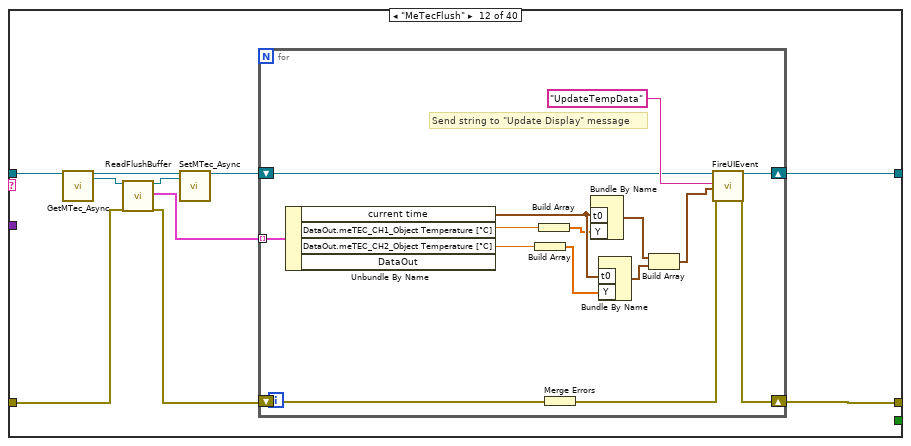
[diagram p17: hidden frame]
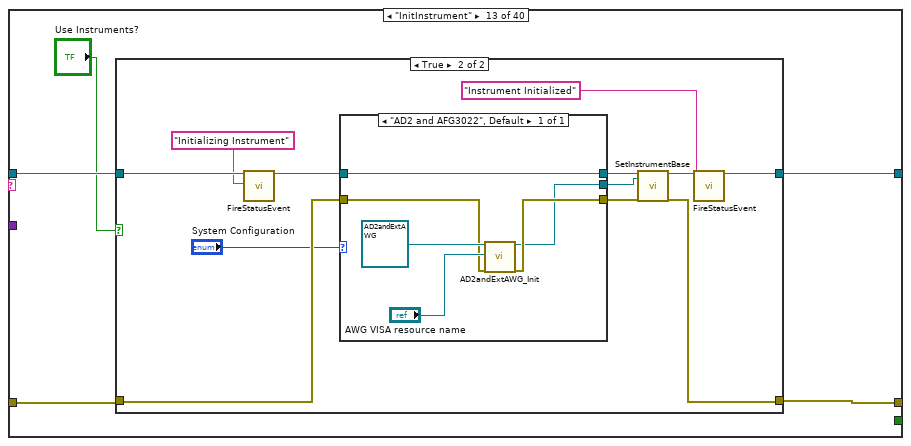
[diagram p18: hidden frame]
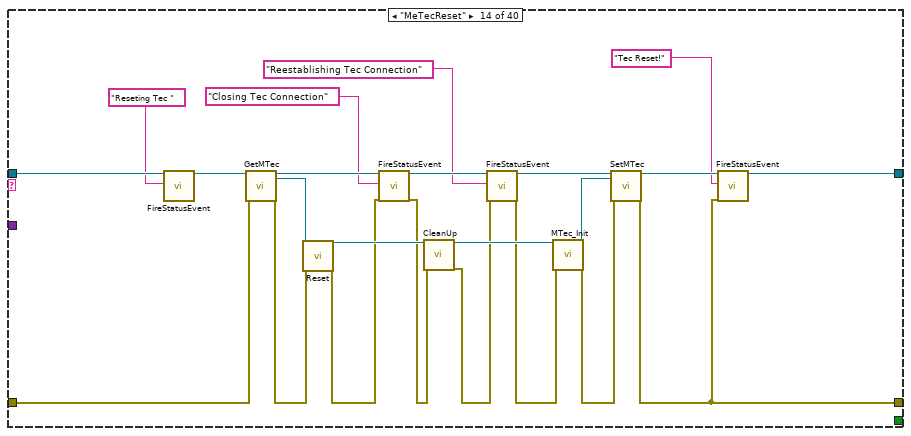
[diagram p20: hidden frame]
diagram:
  (unwired) "AdjustPower" ("Message")
  (unwired) "WfgEnable" ("Message")
  (unwired) "WfgChangeFreq" ("Message")
  # "Save data \nBuild Epxeriment\nSet path\nSave Async Temp Data"
  n1 = local write "OutputEnable"(T13 {"Enable Output WFG Ch1"=FALSE, "Enable Output WFG Ch 2"=FALSE} ("OutputEnable")) -> ()
  n2 = local write "Configdatastd"(T15 {"ConfigDataCh1"={"Frequency Hz (1000 Hz)"=1000.0, "Waveform Function (0: Sine)"=0, "Amplitude (1 Vpp)"=1.0, "DC Offset (0.00 V)"=0.0, "Phase Level (-1)"=0.0, "Phase Unit (0: Radian)"=0}, "ConfigDataCh2"={"Frequency Hz (1000 Hz)"=1000.0, "Waveform Function (0: Sine)"=0, "Amplitude (1 Vpp)"=1.0, "DC Offset (0.00 V)"=0.0, "Phase Level (-1)"=0.0, "Phase Unit (0: Radian)"=0}} ("Configdatastd")) -> ()
  n3 = call "Application_Init.vi"("object in"=refnum<class "Application.lvclass"> refnum ("Application")) -> ("object out"=w12:refnum<class "Application.lvclass">, "error out"=w1:errorcluster)  [unwired: 17 in]
  n4 = call-dynamic "RegisterEvents.vi"("object in"=w12, "error in (no error)"=w1) -> ("object out"=w4:refnum<class "Application.lvclass">, "Event Registration Refnum"=w14:refnum<event-registration>, "error out"=w13:errorcluster)  [unwired: 15 in]
  n5 = property on="Waveform Chart" class="WFChart (strict)"(error in=w1, "History Data"=waveform(dbl)[][] []) -> ()  [unwired: 1 in, 2 out]
  n6 = call-dynamic "FireStatusEvent.vi"("object in"=w4, "Status"="System Not Initialized") -> ()  [unwired: 16 in, 2 out]
  n7 = while {
    tunnel: w1 -> [w16]
    tunnel: [w20] -> w10
    shift-right: [w19] -> w11
    shift-left: w12 -> [w25]
    stop <- w26 stop-if-true
    # "Message Handling Loop"
    n8 = call-dynamic "DeQueueMain.vi"("object in"=w25, "error in (no error)"=w16) -> ("object out"=w24:refnum<class "Application.lvclass">, "Message"=w23:string, "Message Data"=w22:variant, "error out"=w17:errorcluster)  [unwired: 14 in]
    n9 = case "Message Cases" shown="\"MeTecInit\"" w23 {
      selector: w23 -> [_ _ _ _ _ _ _ _ _ _ _ _ _ _ _ _ _ _ _ _ _ _ _ _ _ _ _ _ _ _ _ _ _ _ _ _ _ _ _ w712]
      tunnel: w17 -> [w29 w30 w42 w45 w63 w74 w97 w162 w178 w198 w211 w240 w263 w303 w311 w318 w344 w381 w417 w454 w465 w474 w479 w502 w515 w528 w537 w549 w562 w568 w603 w622 w628 w639 w653 w667 w681 w701 w708 _]
      tunnel: [w28 w35 w37 w53 w64 w76 w98 w162 w180 w206 w228 w244 w262 w285 w310 w316 w349 w385 w414 w455 w464 w475 w488 w505 w516 w529 w538 w550 w563 w569 w604 w623 w634 w647 w660 w672 w676 w689 w707 w713] -> w21
      tunnel: [_ _ _ TRUE _ _ _ _ _ _ _ _ _ _ _ _ _ _ _ _ _ _ _ _ _ _ _ _ _ _ _ _ _ _ _ _ _ _ _ _] -> w26
      tunnel: w22 -> [_ _ w41 w50 _ _ _ _ _ _ _ _ _ _ _ _ _ _ _ _ _ _ w483 w504 _ _ _ _ _ _ w598 w621 w630 w641 w655 w666 _ _ _ _]
      tunnel: w24 -> [w27 w32 w36 w48 w58 w72 w101 w161 w189 w204 w225 w241 w264 w307 w312 w323 w338 w384 w427 w459 w467 w477 w490 w507 w518 w531 w540 w552 w565 w571 w606 w625 w637 w650 w663 w675 w688 w706 w710 w711]
      tunnel: [w27 w33 w36 w49 w65 w71 w100 w160 w176 w202 w208 w237 w261 w289 w309 w326 w353 w386 w426 w457 w466 w476 w489 w506 w517 w521 w539 w544 w564 w570 w602 w624 w627 w648 w661 w665 w680 w700 w709 w711] -> w18
      frame "---Copy This Frame---" {
        # "Duplicate this frame when creating new messages.  Change this comment in the duplicated frame to describe this message."
        n10 = Merge Errors(w29) -> (w28:errorcluster)
      }
      frame "Confirm Quit" {
        # "#CodeNeeded - If you want to provide an \"Are you sure\" dialog (or some other notification) before the application exits, place that code here. This message is typically sent from a Panel Close? event."
        # "Confirm Quit - Message that can confirm whether or not the user wants to exit the application."
        n11 = call-dynamic "EnqueueMain.vi"("object in"=w32, "Message"="Exit", "Message Data"=w30, "error in (no error)"=w30, "Priority Message? (F)"=TRUE) -> ("object out"=w33:refnum<class "Application.lvclass">, "error out"=w35:errorcluster)  [unwired: 13 in]
      }
      frame "Error" {
        # "#CodeRecommended - If you ever change the name of this \"Error\" message, you'll need to update the name in the Check Loop Error.vi as well."
        # "#CodeRecommended - Consider creating a system for logging errors in some way. These errors are for notification purposes only. Handling of specific errors should be performed in the message frames that generated the error."
        # "Error - Display an error dialog. This message is sent by the \"Error Handler\" VIs at the end of other loops in this application."
        n12 = Variant To Data(error in=w42, type=errorcluster {"status"=FALSE, "code"=0, "source"=""} ("error constant"), Variant=w41) -> (data=w39:errorcluster, error out=w38:errorcluster)
        n13 = call <vilib>:"Simple Error Handler.vi"("error in (no error)"=w39) -> ()  [unwired: 4 in, 5 out]
        n14 = Merge Errors(w38) -> (w37:errorcluster)
      }
      frame "Exit" {
        # "Stop the VI"
        # "Release the message queue reference"
        # "#CodeNeeded - Add any required cleanup code here. Note that if 'Exit' was called as a result of an error, an error dialog will be displayed. Add any custom error handling for an 'Exit' condition here as well."
        # "Exit - Exit the application."
        n15 = Variant To Data(error in=w45, type=errorcluster {"status"=FALSE, "code"=0, "source"=""} ("error constant"), Variant=w50) -> (data=w51:errorcluster, error out=w46:errorcluster)
        n16 = call <vilib>:"Simple Error Handler.vi"("error in (no error)"=w51) -> ()  [unwired: 4 in, 5 out]
        n17 = call-dynamic "FireStatusEvent.vi"("object in"=w48, "Status"="Exiting..") -> ("object out"=w44:refnum<class "Application.lvclass">)  [unwired: 16 in, 1 out]
        n18 = call-dynamic "FireStopEvent.vi"("object in"=w44) -> ("object out"=w49:refnum<class "Application.lvclass">, "error out"=w47:errorcluster)  [unwired: 17 in]
        n19 = Merge Errors(w46, w47) -> (w53:errorcluster)
      }
      frame "Initialize" {
        # "Initialize - All initialization work should take place in this message, since other loops can potentially enqueue messages that execute immediately after this one."
        n20 = call-dynamic "FireStatusEvent.vi"("object in"=w58, "Status"="Initializing System") -> ("object out"=w59:refnum<class "Application.lvclass">)  [unwired: 16 in, 1 out]
        n21 = Build Array("MeTecInit" ("Message"), "InitInstrument" ("Message"), "HamamatsuInit" ("Message"), "CetoniInit" ("Message")) -> (w62:string[])
        n22 = for {
          shift-right: [w70] -> w65
          shift-left: w59 -> [w69]
          shift-right: [w68] -> w64
          shift-left: w63 -> [w67]
          tunnel: w62 -> [w66] mode=indexing
          n23 = call-dynamic "EnqueueMain.vi"("object in"=w69, "Message"=w66, "error in (no error)"=w67) -> ("object out"=w70:refnum<class "Application.lvclass">, "error out"=w68:errorcluster)  [unwired: 15 in]
        }
      }
      frame "MeTecInit" {
        # "Something - Replace this message with functionality for your own application."
        n24 = case shown="False" "Use MeTEC?" {
          tunnel: [w84 w95] -> w75
          tunnel: w74 -> [w84 w96]
          tunnel: w72 -> [w78 w90]
          tunnel: [w79 w86] -> w71
          frame False {
            n25 = call-dynamic "FireStatusEvent.vi"("object in"=w78, "Status"="Initializing Dummy") -> ("object out"=w82:refnum<class "Application.lvclass">)  [unwired: 16 in, 1 out]
            n26 = call-dynamic "SetMTec_Async.vi"("object in"=w82, "MTec_Async"=refnum<class "Dummy_Mtec.lvclass"> refnum ("Dummy_Mtec")) -> ("object out"=w81:refnum<class "Application.lvclass">)  [unwired: 16 in, 1 out]
            n27 = call-dynamic "FireStatusEvent.vi"("object in"=w81, "Status"="Dummy Initialized") -> ("object out"=w79:refnum<class "Application.lvclass">)  [unwired: 16 in, 1 out]
          }
          frame True {
            w93 = 1.0  # Sample Rate (Hz)
            n28 = call-dynamic "FireStatusEvent.vi"("object in"=w90, "Status"="Initializing TEC") -> ("object out"=w88:refnum<class "Application.lvclass">)  [unwired: 16 in, 1 out]
            n29 = call "MTEC_Async_Init.vi"("object in"=refnum<class "MTEC_Async.lvclass"> refnum, "SW Buffer Size"=10000, "error in (no error)"=w96, "Sample Rate (Hz)"=w93) -> ("object out"=w92:refnum<class "MTEC_Async.lvclass">, "error out"=w95:errorcluster)  [unwired: 14 in]
            n30 = call-dynamic "SetMTec_Async.vi"("object in"=w88, "MTec_Async"=w92) -> ("object out"=w87:refnum<class "Application.lvclass">)  [unwired: 16 in, 1 out]
            n31 = call-dynamic "FireStatusEvent.vi"("object in"=w87, "Status"="TEC Initialized") -> ("object out"=w86:refnum<class "Application.lvclass">)  [unwired: 16 in, 1 out]
          }
        }
        n32 = Merge Errors(w75) -> (w76:errorcluster)
      }
      frame "HamamatsuInit" {
        n33 = case shown="False" "Use Hamamatsu" {
          tunnel: w101 -> [w103 w133]
          tunnel: [w103 w126] -> w100
          tunnel: [w102 w107] -> w98
          tunnel: w97 -> [w102 w106]
          frame False {
          }
          frame True {
            n34 = call-dynamic "FireStatusEvent.vi"("object in"=w133, "Status"="Init Camera ", "error in (no error)"=w106) -> ("object out"=w128:refnum<class "Application.lvclass">, "error out"=w105:errorcluster)  [unwired: 15 in]
            n35 = call-dynamic "GetHamamatsu.vi"("object in"=w128, "error in (no error)"=w105) -> ("object out"=w132:refnum<class "Application.lvclass">, "Hamamatsu"=w131:refnum<class "Hamamatsu.lvclass">, "error out"=w104:errorcluster)  [unwired: 15 in]
            n36 = call "Hamamatsu_Init.vi"("object in"=w131, "error in (no error)"=w104) -> ("object out"=w130:refnum<class "Hamamatsu.lvclass">, "error out"=w124:errorcluster)  [unwired: 16 in]
            n37 = call-dynamic "OpenCamera.vi"("object in"=w130, "error in (no error)"=w124) -> ("object out"=w116:refnum<class "Hamamatsu.lvclass">, "error out"=w110:errorcluster)  [unwired: 15 in, 1 out]
            n38 = control-ref of="Sub Region"() -> (w114:refnum<vi>)
            n39 = call-dynamic "ReadSubregionLimitsandValue.vi"("object in"=w116, "error in (no error)"=w110) -> ("object out"=w113:refnum<class "Hamamatsu.lvclass">, "Sub Region"=w115:T24, "error out"=w109:errorcluster)  [unwired: 15 in]
            n40 = call-dynamic "UpdateRoiLimits.vi"("object in"=w113, "reference to front panel item"=w114, "SubRegionLimits"=w115, "error in (no error)"=w109) -> ("object out"=w112:refnum<class "Hamamatsu.lvclass">, "error out"=w111:errorcluster)  [unwired: 14 in]
            n41 = call-dynamic "ConfigureSnapshot.vi"("object in"=w112, "error in (no error)"=w111) -> ("object out"=w122:refnum<class "Hamamatsu.lvclass">, "error out"=w123:errorcluster)  [unwired: 16 in]
            n42 = call-dynamic "ConfigureExposureTime.vi"("object in"=w122, "ExposureTime(ms)"=50.0, "error in (no error)"=w123) -> ("object out"=w120:refnum<class "Hamamatsu.lvclass">, "error out"=w119:errorcluster)  [unwired: 15 in]
            n43 = call-dynamic "StartCapture.vi"("object in"=w120, "error in (no error)"=w119) -> ("object out"=w118:refnum<class "Hamamatsu.lvclass">, "error out"=w117:errorcluster)  [unwired: 16 in]
            n44 = call-dynamic "SetHamamatsu.vi"("object in"=w132, "Hamamatsu"=w118, "error in (no error)"=w117) -> ("object out"=w129:refnum<class "Application.lvclass">, "error out"=w108:errorcluster)  [unwired: 15 in]
            n45 = call-dynamic "FireStatusEvent.vi"("object in"=w129, "Status"="Camera Initialized", "error in (no error)"=w108) -> ("object out"=w126:refnum<class "Application.lvclass">, "error out"=w107:errorcluster)  [unwired: 15 in]
          }
        }
      }
      frame "HamamatsuConfigure" {
        n46 = call-dynamic "FireStatusEvent.vi"("object in"=w161, "Status"="Configuring Camera ") -> ("object out"=w157:refnum<class "Application.lvclass">)  [unwired: 16 in, 1 out]
        n47 = call-dynamic "GetHamamatsu.vi"("object in"=w157) -> ("object out"=w159:refnum<class "Application.lvclass">, "Hamamatsu"=w147:refnum<class "Hamamatsu.lvclass">)  [unwired: 16 in, 1 out]
        n48 = call-dynamic "StopCapture.vi"("object in"=w147) -> ("object out"=w146:refnum<class "Hamamatsu.lvclass">, "error out"=w145:errorcluster)  [unwired: 17 in]
        n49 = control-ref of="Sub Region"() -> (w141:refnum<vi>)
        n50 = call-dynamic "ConfigureROI.vi"("object in"=w146, "Sub Region"="ROI", "error in (no error)"=w145) -> ("object out"=w143:refnum<class "Hamamatsu.lvclass">, "SubRegionLimits"=w140:T25, "error out"=w142:errorcluster)  [unwired: 14 in]
        n51 = case shown="True" "Center ROI" {
          tunnel: w143 -> [w163 w170]
          tunnel: [w163 w169] -> w139
          tunnel: w142 -> [w164 w168]
          tunnel: [w164 w167] -> w137
          tunnel: w140 -> [w165 _]
          tunnel: [w165 w166] -> w135
          frame False {
          }
          frame True {
            n52 = call-dynamic "CenterROI.vi"("object in"=w170, "error in (no error)"=w168) -> ("object out"=w169:refnum<class "Hamamatsu.lvclass">, "Sub Region"=w166:T24, "error out"=w167:errorcluster)  [unwired: 15 in]
          }
        }
        n53 = call-dynamic "UpdateRoiLimits.vi"("object in"=w139, "reference to front panel item"=w141, "SubRegionLimits"=w135, "error in (no error)"=w137) -> ("object out"=w138:refnum<class "Hamamatsu.lvclass">, "error out"=w136:errorcluster)  [unwired: 14 in]
        n54 = call-dynamic "ConfigureSnapshot.vi"("object in"=w138, "error in (no error)"=w136) -> ("object out"=w153:refnum<class "Hamamatsu.lvclass">, "error out"=w154:errorcluster)  [unwired: 16 in]
        n55 = call-dynamic "ConfigureExposureTime.vi"("object in"=w153, "ExposureTime(ms)"="ExposureTime(ms)", "error in (no error)"=w154) -> ("object out"=w151:refnum<class "Hamamatsu.lvclass">, "error out"=w150:errorcluster)  [unwired: 15 in]
        n56 = call-dynamic "StartCapture.vi"("object in"=w151, "error in (no error)"=w150) -> ("object out"=w149:refnum<class "Hamamatsu.lvclass">, "error out"=w148:errorcluster)  [unwired: 16 in]
        n57 = call-dynamic "SetHamamatsu.vi"("object in"=w159, "Hamamatsu"=w149, "error in (no error)"=w148) -> ("object out"=w158:refnum<class "Application.lvclass">)  [unwired: 15 in, 1 out]
        n58 = call-dynamic "FireStatusEvent.vi"("object in"=w158, "Status"="CameraConfigured") -> ("object out"=w160:refnum<class "Application.lvclass">)  [unwired: 16 in, 1 out]
      }
      frame "HamamatsuImage" {
        n59 = call-dynamic "FireStatusEvent.vi"("object in"=w189, "Status"="Imaging", "error in (no error)"=w178) -> ("object out"=w186:refnum<class "Application.lvclass">, "error out"=w179:errorcluster)  [unwired: 15 in]
        n60 = call-dynamic "GetHamamatsu.vi"("object in"=w186, "error in (no error)"=w179) -> ("object out"=w188:refnum<class "Application.lvclass">, "Hamamatsu"=w184:refnum<class "Hamamatsu.lvclass">, "error out"=w177:errorcluster)  [unwired: 15 in]
        n61 = call-dynamic "CaptureSnapshot.vi"("object in"=w184, "error in (no error)"=w177) -> ("object out"=w183:refnum<class "Hamamatsu.lvclass">, "FreeRunningImage"=w182:T26, "error out"=w181:errorcluster)  [unwired: 14 in, 1 out]
        n62 = call "IMAQ WindDraw"("Resize to Image Size? (Y)"=FALSE, "error in (no error)"=w181, "Image"=w182) -> ("error out"=w172:errorcluster)  [unwired: 7 in, 1 out]
        n63 = call-dynamic "SetHamamatsu.vi"("object in"=w188, "Hamamatsu"=w183, "error in (no error)"=w172) -> ("object out"=w187:refnum<class "Application.lvclass">, "error out"=w180:errorcluster)  [unwired: 15 in]
        n64 = call "IMAQ WindZoom 2"("error in (no error)"=w172, "Zoom to Fit? (False)"=TRUE) -> ()  [unwired: 6 in, 4 out]
        n65 = case shown="False" "Image Continous" {
          tunnel: w187 -> [w190 w193]
          tunnel: [w190 w192] -> w176
          tunnel: "HamamatsuImage" ("Message") -> [_ w191]
          frame False {
          }
          frame True {
            n66 = call-dynamic "EnqueueMain.vi"("object in"=w193, "Message"=w191) -> ("object out"=w192:refnum<class "Application.lvclass">)  [unwired: 16 in, 1 out]
          }
        }
      }
      frame "MeTecConfigure" {
        # "Send string to \"Update Display\" message"
        # "Something - Replace this message with functionality for your own application."
        n67 = call-dynamic "FireStatusEvent.vi"("object in"=w204, "Status"="Configuring TEC") -> ("object out"=w200:refnum<class "Application.lvclass">)  [unwired: 16 in, 1 out]
        n68 = call-dynamic "GetMTec_Async.vi"("object in"=w200) -> ("object out"=w203:refnum<class "Application.lvclass">, "MTec_Async"=w196:refnum<class "MTEC_Async.lvclass">)  [unwired: 16 in, 1 out]
        n69 = call-dynamic "Configure.vi"("object in"=w196, "Config Data"="Config Data", "error in (no error)"=w198) -> ("object out"=w195:refnum<class "MTEC_Async.lvclass">, "error out"=w197:errorcluster)  [unwired: 15 in]
        n70 = call-dynamic "SetMTec_Async.vi"("object in"=w203, "MTec_Async"=w195) -> ("object out"=w205:refnum<class "Application.lvclass">)  [unwired: 16 in, 1 out]
        n71 = Merge Errors(w197) -> (w206:errorcluster)
        n72 = call-dynamic "FireStatusEvent.vi"("object in"=w205, "Status"="TEC Configured") -> ("object out"=w202:refnum<class "Application.lvclass">)  [unwired: 16 in, 1 out]
      }
      frame "MeTecMonitor" {
        # "Send string to \"Update Display\" message"
        # "Something - Replace this message with functionality for your own application."
        n73 = call-dynamic "GetMTec_Async.vi"("object in"=w225) -> ("object out"=w226:refnum<class "Application.lvclass">, "MTec_Async"=w215:refnum<class "MTEC_Async.lvclass">)  [unwired: 16 in, 1 out]
        n74 = call-dynamic "ForceAndReadNew.vi"("object in"=w215, "Buffer Values"=TRUE, "error in (no error)"=w211) -> ("object out"=w214:refnum<class "MTEC_Async.lvclass">, "Cluster"=w213:T27, "error out"=w212:errorcluster)  [unwired: 14 in]
        n75 = Unbundle By Name(w213) -> ("current time"=w220:timestamp, "DataOut.meTEC_CH1_Object Temperature [°C]"=w224:dbl, "DataOut.meTEC_CH2_Object Temperature [°C]"=w217:dbl, "DataOut"=→"Cluster":T8)
        n76 = call-dynamic "SetMTec_Async.vi"("object in"=w226, "MTec_Async"=w214) -> ("object out"=w227:refnum<class "Application.lvclass">)  [unwired: 16 in, 1 out]
        n77 = Build Array(w217) -> (w216:dbl[])
        n78 = Build Array(w224) -> (w219:dbl[])
        n79 = Bundle By Name("t0"=w220, "Y"=w219) -> (w222:waveform(dbl))  [unwired: 1 in]
        n80 = Bundle By Name("t0"=w220, "Y"=w216) -> (w221:waveform(dbl))  [unwired: 1 in]
        n81 = Merge Errors(w212) -> (w229:errorcluster)
        n82 = local read "Monitor"() -> (w207:bool)
        n83 = Build Array(w222, w221) -> (w218:waveform(dbl)[])
        n84 = call-dynamic "FireUIEvent.vi"("object in"=w227, "Message"="UpdateTempData", "Message Data"=w218, "error in (no error)"=w229) -> ("object out"=w209:refnum<class "Application.lvclass">, "error out"=w228:errorcluster)  [unwired: 14 in]
        n85 = case shown="True" w207 {
          tunnel: w209 -> [w231 w233]
          tunnel: [w231 w232] -> w208
          frame False {
          }
          frame True {
            n86 = call-dynamic "EnqueueMain.vi"("object in"=w233, "Message"="MeTecMonitor") -> ("object out"=w232:refnum<class "Application.lvclass">)  [unwired: 16 in, 1 out]
          }
        }
      }
      frame "MeTecFlush" {
        # "Something - Replace this message with functionality for your own application."
        n87 = call-dynamic "GetMTec_Async.vi"("object in"=w241) -> ("object out"=w242:refnum<class "Application.lvclass">, "MTec_Async"=w238:refnum<class "MTEC_Async.lvclass">)  [unwired: 16 in, 1 out]
        n88 = call-dynamic "ReadFlushBuffer.vi"("object in"=w238, "error in (no error)"=w240) -> ("object out"=w236:refnum<class "MTEC_Async.lvclass">, "Stored Data"=w235:T28, "error out"=w239:errorcluster)  [unwired: 15 in]
        n89 = call-dynamic "SetMTec_Async.vi"("object in"=w242, "MTec_Async"=w236) -> ("object out"=w243:refnum<class "Application.lvclass">)  [unwired: 16 in, 1 out]
        n90 = for {
          tunnel: w235 -> [w245] mode=indexing
          shift-right: [w246] -> w237
          shift-left: w243 -> [w256]
          shift-right: [w257] -> w244
          shift-left: w239 -> [w247]
          # "Send string to \"Update Display\" message"
          n91 = Unbundle By Name(w245) -> ("current time"=w252:timestamp, "DataOut.meTEC_CH1_Object Temperature [°C]"=w255:dbl, "DataOut.meTEC_CH2_Object Temperature [°C]"=w249:dbl)  [unwired: 1 out]
          n92 = Build Array(w249) -> (w248:dbl[])
          n93 = Build Array(w255) -> (w251:dbl[])
          n94 = Merge Errors(w247) -> (w258:errorcluster)
          n95 = Bundle By Name("t0"=w252, "Y"=w251) -> (w254:waveform(dbl))  [unwired: 1 in]
          n96 = Bundle By Name("t0"=w252, "Y"=w248) -> (w253:waveform(dbl))  [unwired: 1 in]
          n97 = Build Array(w254, w253) -> (w250:waveform(dbl)[])
          n98 = call-dynamic "FireUIEvent.vi"("object in"=w256, "Message"="UpdateTempData", "Message Data"=w250, "error in (no error)"=w258) -> ("object out"=w246:refnum<class "Application.lvclass">, "error out"=w257:errorcluster)  [unwired: 14 in]
        }
      }
      frame "InitInstrument" {
        n99 = case shown="True" "Use Instruments?" {
          tunnel: w264 -> [w266 w278]
          tunnel: w263 -> [w265 w277]
          tunnel: [w265 w273] -> w262
          tunnel: [w266 w268] -> w261
          frame False {
          }
          frame True {
            n100 = call-dynamic "FireStatusEvent.vi"("object in"=w278, "Status"="Initializing Instrument") -> ("object out"=w270:refnum<class "Application.lvclass">)  [unwired: 16 in, 1 out]
            n101 = case shown="\"AD2 and AFG3022\", Default" "System Configuration" {
              tunnel: w270 -> [w280]
              tunnel: w277 -> [w282]
              tunnel: [w281] -> w275
              tunnel: [w280] -> w272
              tunnel: [w279] -> w271
              frame "AD2 and AFG3022", Default {
                n102 = call "AD2andExtAWG_Init.vi"("object in"=refnum<class "AD2andExtAWG.lvclass"> refnum ("AD2andExtAWG"), "VISA resource name"="AWG VISA resource name", "error in (no error)"=w282) -> ("object out"=w279:refnum<class "AD2andExtAWG.lvclass">, "error out"=w281:errorcluster)  [unwired: 15 in]
              }
            }
            n103 = call-dynamic "SetInstrumentBase.vi"("object in"=w272, "InstrumentBase"=w271, "error in (no error)"=w275) -> ("object out"=w274:refnum<class "Application.lvclass">, "error out"=w273:errorcluster)  [unwired: 15 in]
            n104 = call-dynamic "FireStatusEvent.vi"("object in"=w274, "Status"="Instrument Initialized") -> ("object out"=w268:refnum<class "Application.lvclass">)  [unwired: 16 in, 1 out]
          }
        }
      }
      frame "MeTecReset" {
        n105 = call-dynamic "FireStatusEvent.vi"("object in"=w307, "Status"="Reseting Tec ") -> ("object out"=w301:refnum<class "Application.lvclass">)  [unwired: 16 in, 1 out]
        n106 = call-dynamic "GetMTec.vi"("object in"=w301, "error in (no error)"=w303) -> ("object out"=w306:refnum<class "Application.lvclass">, "MTec"=w304:refnum<class "MTec.lvclass">, "error out"=w302:errorcluster)  [unwired: 15 in]
        n107 = call-dynamic "Reset.vi"("object in"=w304, "error in (no error)"=w302) -> ("object out"=w300:refnum<class "MTec.lvclass">, "error out"=w292:errorcluster)  [unwired: 16 in]
        n108 = call-dynamic "FireStatusEvent.vi"("object in"=w306, "Status"="Closing Tec Connection", "error in (no error)"=w292) -> ("object out"=w297:refnum<class "Application.lvclass">, "error out"=w291:errorcluster)  [unwired: 15 in]
        n109 = call-dynamic "CleanUp.vi"("object in"=w300, "error in (no error)"=w291) -> ("object out"=w299:refnum<class "MTec.lvclass">, "error out"=w293:errorcluster)  [unwired: 16 in]
        n110 = call-dynamic "FireStatusEvent.vi"("object in"=w297, "Status"="Reestablishing Tec Connection", "error in (no error)"=w293) -> ("object out"=w296:refnum<class "Application.lvclass">, "error out"=w295:errorcluster)  [unwired: 15 in]
        n111 = call "MTec_Init.vi"("object in"=w299, "error in (no error)"=w295) -> ("object out"=w298:refnum<class "MTec.lvclass">, "error out"=w294:errorcluster)  [unwired: 16 in]
        n112 = call-dynamic "SetMTec.vi"("object in"=w296, "MTec"=w298, "error in (no error)"=w294) -> ("object out"=w305:refnum<class "Application.lvclass">, "error out"=w285:errorcluster)  [unwired: 15 in]
        n113 = call-dynamic "FireStatusEvent.vi"("object in"=w305, "Status"="Tec Reset!", "error in (no error)"=w285) -> ("object out"=w289:refnum<class "Application.lvclass">)  [unwired: 15 in, 1 out]
      }
      frame "Abort" {
        # "Might have to close fileref here etc.."
        n114 = call-dynamic "FlushMainQueue.vi"("object in"=w312, "error in (no error)"=w311) -> ("object out"=w313:refnum<class "Application.lvclass">, "error out"=w310:errorcluster)  [unwired: 15 in, 1 out]
        n115 = call-dynamic "FireStatusEvent.vi"("object in"=w313, "Status"="Sequence Aborted") -> ("object out"=w309:refnum<class "Application.lvclass">)  [unwired: 16 in, 1 out]
      }
      frame "StartPwrScan" {
        n116 = call-dynamic "GetInstrumentBase.vi"("object in"=w323, "error in (no error)"=w318) -> ("object out"=w325:refnum<class "Application.lvclass">, "InstrumentBase"=w322:refnum<class "InstrumentBase.lvclass">, "error out"=w319:errorcluster)  [unwired: 15 in]
        n117 = call-dynamic "StartPowerScan.vi"("object in"=w322, "PwrScanSettings"="PwrScanSettings", "CurrentProbeScaling(V/A)"="CurrentProbeScaling(V/A)", "error in (no error)"=w319) -> ("object out"=w321:refnum<class "InstrumentBase.lvclass">, "error out"=w317:errorcluster)  [unwired: 14 in]
        n118 = call-dynamic "SetInstrumentBase.vi"("object in"=w325, "InstrumentBase"=w321, "error in (no error)"=w317) -> ("object out"=w324:refnum<class "Application.lvclass">, "error out"=w316:errorcluster)  [unwired: 15 in]
        n119 = call-dynamic "EnqueueMain.vi"("object in"=w324, "Message"="RunPwrScan") -> ("object out"=w326:refnum<class "Application.lvclass">)  [unwired: 16 in, 1 out]
      }
      frame "StartExperiment" {
        n120 = call-dynamic "GetExperiment.vi"("object in"=w338) -> ("object out"=w339:refnum<class "Application.lvclass">, "Experiment"=w337:refnum<class "Experiment.lvclass">)  [unwired: 16 in, 1 out]
        n121 = call "Experiment_Init.vi"("object in"=w337, "error in (no error)"=w344) -> ("object out"=w346:refnum<class "Experiment.lvclass">, "error out"=w345:errorcluster)  [unwired: 16 in]
        n122 = call-dynamic "BuildExperiment.vi"("object in"=w346, "List of Frequencies"="List of Frequencies (Hz)", "List of Powers to run(W)"="List of Powers to run(W)", "Number of Images"="Number of Images (#)", "wait time(s)"="wait time(s)", "error in (no error)"=w345, "AutoRange MSO"="AutoRange MSO", "Flow"="List of Flow Rates (ul/min)", "wait after changing flow rate(s)"="wait after changing flow rate(s)", "Repeat Adjust Power and Wait N Times"="Repeat Adjust Power and Wait N Times (#)", "wait after adjust power"="wait after adjust power (s)") -> ("object out"=w342:refnum<class "Experiment.lvclass">, "# elements in queue"=→"# elements in queue":i32, "error out"=w341:errorcluster)  [unwired: 6 in]
        n123 = call-dynamic "SetExperiment.vi"("object in"=w339, "Experiment"=w342, "error in (no error)"=w341) -> ("object out"=w343:refnum<class "Application.lvclass">, "error out"=w340:errorcluster)  [unwired: 15 in]
        n124 = call-dynamic "GetTDMSLloggPWR.vi"("object in"=w343) -> ("object out"=w351:refnum<class "Application.lvclass">, "TDMSLloggPWR"=w352:refnum<class "TDMSLogger_PowerScan.lvclass">)  [unwired: 16 in, 1 out]
        n125 = call "TDMSLogger_PowerScan_Init.vi"("object in"=w352, "error in (no error)"=w340) -> ("object out"=w347:refnum<class "TDMSLogger_PowerScan.lvclass">, "cancelled"=w350:bool, "error out"=w348:errorcluster)  [unwired: 15 in]
        n126 = case shown="False" w350 {
          tunnel: [w361 w365] -> w353
          tunnel: w351 -> [w359 w366]
          tunnel: [w357 w363] -> w349
          tunnel: w348 -> [w356 w364]
          tunnel: w347 -> [w355 _]
          frame False {
            n127 = call-dynamic "SetTDMSLloggPWR.vi"("object in"=w359, "TDMSLloggPWR"=w355, "error in (no error)"=w356) -> ("object out"=w360:refnum<class "Application.lvclass">, "error out"=w358:errorcluster)  [unwired: 15 in]
            n128 = call-dynamic "EnqueueMain.vi"("object in"=w360, "Message"="RunExperiment", "error in (no error)"=w358) -> ("object out"=w361:refnum<class "Application.lvclass">, "error out"=w357:errorcluster)  [unwired: 15 in]
          }
          frame True {
            n129 = call-dynamic "FireStatusEvent.vi"("object in"=w366, "Status"="Experiment Complete", "error in (no error)"=w364) -> ("object out"=w365:refnum<class "Application.lvclass">, "error out"=w363:errorcluster)  [unwired: 15 in]
          }
        }
      }
      frame "RunExperiment" {
        n130 = local read "# elements in queue"() -> (w372:i32)
        n131 = call-dynamic "GetExperiment.vi"("object in"=w384) -> ("object out"=w379:refnum<class "Application.lvclass">, "Experiment"=w383:refnum<class "Experiment.lvclass">)  [unwired: 16 in, 1 out]
        n132 = call-dynamic "DequeueExperiment.vi"("object in"=w383, "error in (no error)"=w381) -> ("# elements in queue"=w373:i32, "object out"=w380:refnum<class "Experiment.lvclass">, "Message"=w375:string, "Message Data"=w374:variant, "QueueEmpty"=w382:bool, "error out"=w377:errorcluster)  [unwired: 12 in]
        n133 = call-dynamic "SetExperiment.vi"("object in"=w379, "Experiment"=w380, "error in (no error)"=w377) -> ("object out"=w378:refnum<class "Application.lvclass">, "error out"=w376:errorcluster)  [unwired: 15 in]
        n134 = Divide(x=w373, y=w372) -> (x/y=w371:dbl)
        n135 = Subtract(x=1.0, y=w371) -> (x-y=w369:dbl)
        n136 = Multiply(x=w369, y=100.0) -> (x*y=→"Progress (100%)":dbl)
        n137 = case shown="True" w382 {
          tunnel: [w390 w407] -> w386
          tunnel: w378 -> [w395 w403]
          tunnel: [w387 w400] -> w385
          tunnel: w376 -> [w393 w399]
          tunnel: w375 -> [w394 _]
          tunnel: w374 -> [w392 _]
          frame False {
            n138 = call-dynamic "EnqueueMain.vi"("object in"=w395, "Message"=w394, "Message Data"=w392, "error in (no error)"=w393) -> ("object out"=w396:refnum<class "Application.lvclass">, "error out"=w391:errorcluster)  [unwired: 14 in]
            n139 = call-dynamic "EnqueueMain.vi"("object in"=w396, "Message"="RunExperiment", "error in (no error)"=w391) -> ("object out"=w398:refnum<class "Application.lvclass">, "error out"=w388:errorcluster)  [unwired: 15 in]
            n140 = call-dynamic "FireStatusEvent.vi"("object in"=w398, "Status"="Running Experiment", "error in (no error)"=w388) -> ("object out"=w390:refnum<class "Application.lvclass">, "error out"=w387:errorcluster)  [unwired: 15 in]
          }
          frame True {
            n141 = call-dynamic "GetTDMSLloggPWR.vi"("object in"=w403) -> ("object out"=w405:refnum<class "Application.lvclass">, "TDMSLloggPWR"=w402:refnum<class "TDMSLogger_PowerScan.lvclass">)  [unwired: 16 in, 1 out]
            n142 = call-dynamic "CleanUp.vi"("object in"=w402, "error in (no error)"=w399) -> ("object out"=w401:refnum<class "TDMSLogger_PowerScan.lvclass">, "error out"=w400:errorcluster)  [unwired: 16 in]
            n143 = call-dynamic "SetTDMSLloggPWR.vi"("object in"=w405, "TDMSLloggPWR"=w401) -> ("object out"=w404:refnum<class "Application.lvclass">)  [unwired: 16 in, 1 out]
            n144 = call-dynamic "FireStatusEvent.vi"("object in"=w404, "Status"="Experiment Complete") -> ("object out"=w407:refnum<class "Application.lvclass">)  [unwired: 16 in, 1 out]
          }
        }
      }
      frame "RunPwrScan" {
        n145 = call-dynamic "GetInstrumentBase.vi"("object in"=w427, "error in (no error)"=w417) -> ("object out"=w425:refnum<class "Application.lvclass">, "InstrumentBase"=w423:refnum<class "InstrumentBase.lvclass">, "error out"=w416:errorcluster)  [unwired: 15 in]
        n146 = call-dynamic "RunPowerScan.vi"("object in"=w423, "error in (no error)"=w416) -> ("Impedance"=w409:cluster{dbl[], dbl[]}, "Phase"=w408:cluster{dbl[], dbl[]}, "object out"=w422:refnum<class "InstrumentBase.lvclass">, "PowerScanComplete"=w421:bool, "PowerScanResult"=w411:cluster{"PwrFreq":dbl[], "PwrMeasured":dbl[]}, "Channels array"=w415:waveform(dbl)[], "error out"=w413:errorcluster)  [unwired: 11 in]
        n147 = Unbundle By Name(w411) -> ("PwrMeasured"=w420:dbl[])
        n148 = call-dynamic "SetInstrumentBase.vi"("object in"=w425, "InstrumentBase"=w422, "error in (no error)"=w413) -> ("object out"=w424:refnum<class "Application.lvclass">, "error out"=w412:errorcluster)  [unwired: 15 in]
        n149 = Build Array(w411, w409, w408) -> (→"Power Graph":cluster{"PwrFreq":dbl[], "PwrMeasured":dbl[]}[])
        n150 = Array Max & Min(array=w420) -> (max value=→"max Power":dbl, min value=→"min Power":dbl)  [unwired: 2 out]
        n151 = case shown="False" w421 {
          tunnel: [w439 w443] -> w426
          tunnel: w424 -> [w438 w444]
          tunnel: w415 -> [w435 _]
          tunnel: w412 -> [w432 w440]
          tunnel: [w433 w441] -> w414
          frame False {
            n152 = call-dynamic "FireUIEvent.vi"("object in"=w438, "Message"="UpdateMsoData", "Message Data"=w435, "error in (no error)"=w432) -> ("object out"=w436:refnum<class "Application.lvclass">, "error out"=w430:errorcluster)  [unwired: 14 in]
            n153 = call-dynamic "FireStatusEvent.vi"("object in"=w436, "Status"="Running PowerScan", "error in (no error)"=w430) -> ("object out"=w431:refnum<class "Application.lvclass">, "error out"=w429:errorcluster)  [unwired: 15 in]
            n154 = call-dynamic "EnqueueMain.vi"("object in"=w431, "Message"="RunPwrScan", "error in (no error)"=w429) -> ("object out"=w439:refnum<class "Application.lvclass">, "error out"=w433:errorcluster)  [unwired: 15 in]
          }
          frame True {
            n155 = call-dynamic "FireStatusEvent.vi"("object in"=w444, "Status"="PowerScan Complete", "error in (no error)"=w440) -> ("object out"=w443:refnum<class "Application.lvclass">, "error out"=w441:errorcluster)  [unwired: 15 in]
          }
        }
      }
      frame "MeasurePwr" {
        n156 = local read "CurrentProbeScaling(V/A)"() -> (w450:dbl)
        n157 = call-dynamic "GetInstrumentBase.vi"("object in"=w459, "error in (no error)"=w454) -> ("object out"=w458:refnum<class "Application.lvclass">, "InstrumentBase"=w452:refnum<class "InstrumentBase.lvclass">, "error out"=w449:errorcluster)  [unwired: 15 in]
        n158 = call-dynamic "SetCurrentProbeScaling(VA).vi"("object in"=w452, "CurrentProbeScaling(V/A)"=w450, "error in (no error)"=w449) -> ("object out"=w451:refnum<class "InstrumentBase.lvclass">, "error out"=w448:errorcluster)  [unwired: 15 in]
        n159 = call-dynamic "MeasurePower.vi"("object in"=w451, "error in (no error)"=w448) -> ("impedance (ohm)"=→"impedance (ohm)":dbl, "phase (deg)"=→"phase (deg)":dbl, "object out"=w456:refnum<class "InstrumentBase.lvclass">, "Measured Power"=→"Measured Power":dbl, "error out"=w447:errorcluster)  [unwired: 12 in, 1 out]
        n160 = call-dynamic "SetInstrumentBase.vi"("object in"=w458, "InstrumentBase"=w456, "error in (no error)"=w447) -> ("object out"=w457:refnum<class "Application.lvclass">, "error out"=w455:errorcluster)  [unwired: 15 in]
      }
      frame "CetoniCondRefill" {
        n161 = call-dynamic "ConditionalRefill.vi"("object in"=w467, "Turn Off WFG During Refill"="Turn Off WFG During Refill", "refill below level(uL)"="refill below level(uL)", "refill and \nempty rate(uL/min)"="refill and \nempty rate(uL/min)", "error in (no error)"=w465, "Wait After Conditional Refill (s)"="Wait After Conditional Refill (s)") -> ("object out"=w466:refnum<class "Application.lvclass">, "error out"=w464:errorcluster)  [unwired: 12 in]
      }
      frame "CetoniRefill" {
        n162 = call-dynamic "GetCetoniPump.vi"("object in"=w477, "error in (no error)"=w474) -> ("object out"=w478:refnum<class "Application.lvclass">, "CetoniPump"=w473:refnum<class "CetoniPump.lvclass">, "error out"=w471:errorcluster)  [unwired: 15 in]
        n163 = local read "refill and \nempty rate(uL/min)"() -> (w468:dbl)
        n164 = local read "index"() -> (w469:i32)
        n165 = call-dynamic "Refill.vi"("object in"=w473, "refill rate"=w468, "index"=w469, "error in (no error)"=w471) -> ("object out"=w472:refnum<class "CetoniPump.lvclass">, "error out"=w470:errorcluster)  [unwired: 14 in]
        n166 = call-dynamic "SetCetoniPump.vi"("object in"=w478, "CetoniPump"=w472, "error in (no error)"=w470) -> ("object out"=w476:refnum<class "Application.lvclass">, "error out"=w475:errorcluster)  [unwired: 15 in]
      }
      frame "CetoniToggleValve" {
        n167 = Variant To Data(error in=w479, type=cluster{"index":i32, "Valve Position":bool} {"index"=0, "Valve Position"=FALSE} ("ValveControl"), Variant=w483) -> (data=w481:cluster{"index":i32, "Valve Position":bool}, error out=w480:errorcluster)
        n168 = call-dynamic "GetCetoniPump.vi"("object in"=w490, "error in (no error)"=w480) -> ("object out"=w491:refnum<class "Application.lvclass">, "CetoniPump"=w487:refnum<class "CetoniPump.lvclass">, "error out"=w485:errorcluster)  [unwired: 15 in]
        n169 = call-dynamic "ToggleValve.vi"("object in"=w487, "ValveControl"=w481, "error in (no error)"=w485) -> ("object out"=w486:refnum<class "CetoniPump.lvclass">, "error out"=w484:errorcluster)  [unwired: 15 in]
        n170 = call-dynamic "SetCetoniPump.vi"("object in"=w491, "CetoniPump"=w486, "error in (no error)"=w484) -> ("object out"=w489:refnum<class "Application.lvclass">, "error out"=w488:errorcluster)  [unwired: 15 in]
      }
      frame "CetoniGoToLevel" {
        n171 = Variant To Data(error in=w502, type=T22 {"index"=0, "Level(ml)"=0.0, "Flow"=0.0} ("GoToLevelSettings"), Variant=w504) -> (data=w496:T22, error out=w503:errorcluster)
        n172 = call-dynamic "GetCetoniPump.vi"("object in"=w507, "error in (no error)"=w503) -> ("object out"=w508:refnum<class "Application.lvclass">, "CetoniPump"=w501:refnum<class "CetoniPump.lvclass">, "error out"=w500:errorcluster)  [unwired: 15 in]
        n173 = call-dynamic "SetFillLevel.vi"("object in"=w501, "GoToLevelSettings"=w496, "error in (no error)"=w500) -> ("object out"=w498:refnum<class "CetoniPump.lvclass">, "Coerced Level"=w494:dbl, "Coerced Flow"=w493:dbl, "error out"=w499:errorcluster)  [unwired: 12 in, 1 out]
        n174 = call-dynamic "SetCetoniPump.vi"("object in"=w508, "CetoniPump"=w498, "error in (no error)"=w499) -> ("object out"=w506:refnum<class "Application.lvclass">, "error out"=w505:errorcluster)  [unwired: 15 in]
        n175 = local read "GoToLevelSettings"() -> (w495:T4)
        n176 = Bundle By Name(cluster=w495, "Level(uL)"=w494, "Flow"=w493) -> (w492:T4)
        n177 = local write "GoToLevelSettings"(w492) -> ()
      }
      frame "CetoniConfigure" {
        n178 = call-dynamic "GetCetoniPump.vi"("object in"=w518, "error in (no error)"=w515) -> ("object out"=w519:refnum<class "Application.lvclass">, "CetoniPump"=w514:refnum<class "CetoniPump.lvclass">, "error out"=w512:errorcluster)  [unwired: 15 in]
        n179 = local read "index"() -> (w510:i32)
        n180 = call-dynamic "ConfigureSyringe.vi"("object in"=w514, "index"=w510, "SyringeSettings"="SyringeSettings", "error in (no error)"=w512) -> ("object out"=w513:refnum<class "CetoniPump.lvclass">, "error out"=w511:errorcluster)  [unwired: 14 in]
        n181 = call-dynamic "SetCetoniPump.vi"("object in"=w519, "CetoniPump"=w513, "error in (no error)"=w511) -> ("object out"=w517:refnum<class "Application.lvclass">, "error out"=w516:errorcluster)  [unwired: 15 in]
      }
      frame "CetoniRefMove" {
        n182 = call-dynamic "GetCetoniPump.vi"("object in"=w531, "error in (no error)"=w528) -> ("object out"=w522:refnum<class "Application.lvclass">, "CetoniPump"=w527:refnum<class "CetoniPump.lvclass">, "error out"=w525:errorcluster)  [unwired: 15 in]
        n183 = call-dynamic "ReferenceMove.vi"("object in"=w527, "index"=0, "error in (no error)"=w525) -> ("object out"=w526:refnum<class "CetoniPump.lvclass">, "error out"=w524:errorcluster)  [unwired: 15 in]
        n184 = call-dynamic "SetCetoniPump.vi"("object in"=w522, "CetoniPump"=w526, "error in (no error)"=w524) -> ("object out"=w530:refnum<class "Application.lvclass">, "error out"=w529:errorcluster)  [unwired: 15 in]
        n185 = call-dynamic "FireStatusEvent.vi"("object in"=w530, "Status"="Reference Move") -> ("object out"=w521:refnum<class "Application.lvclass">)  [unwired: 16 in, 1 out]
      }
      frame "CetoniEmpty" {
        n186 = call-dynamic "GetCetoniPump.vi"("object in"=w540, "error in (no error)"=w537) -> ("object out"=w541:refnum<class "Application.lvclass">, "CetoniPump"=w536:refnum<class "CetoniPump.lvclass">, "error out"=w534:errorcluster)  [unwired: 15 in]
        n187 = local read "index"() -> (w532:i32)
        n188 = call-dynamic "Empty.vi"("object in"=w536, "index"=w532, "error in (no error)"=w534) -> ("object out"=w535:refnum<class "CetoniPump.lvclass">, "error out"=w533:errorcluster)  [unwired: 15 in]
        n189 = call-dynamic "SetCetoniPump.vi"("object in"=w541, "CetoniPump"=w535, "error in (no error)"=w533) -> ("object out"=w539:refnum<class "Application.lvclass">, "error out"=w538:errorcluster)  [unwired: 15 in]
      }
      frame "CetoniMonitor" {
        n190 = call-dynamic "GetCetoniPump.vi"("object in"=w552, "error in (no error)"=w549) -> ("object out"=w553:refnum<class "Application.lvclass">, "CetoniPump"=w548:refnum<class "CetoniPump.lvclass">, "error out"=w546:errorcluster)  [unwired: 15 in]
        n191 = call-dynamic "ReadStatusAllPumps.vi"("object in"=w548, "error in (no error)"=w546) -> ("object out"=w547:refnum<class "CetoniPump.lvclass">, "Array"=→"Array":T5, "error out"=w545:errorcluster)  [unwired: 15 in]
        n192 = local read "Monitor Pump"() -> (w543:bool)
        n193 = call-dynamic "SetCetoniPump.vi"("object in"=w553, "CetoniPump"=w547, "error in (no error)"=w545) -> ("object out"=w551:refnum<class "Application.lvclass">, "error out"=w550:errorcluster)  [unwired: 15 in]
        n194 = case shown="False" w543 {
          tunnel: w551 -> [w554 w557]
          tunnel: [w554 w556] -> w544
          frame False {
          }
          frame True {
            n195 = call-dynamic "EnqueueMain.vi"("object in"=w557, "Message"="CetoniMonitor") -> ("object out"=w556:refnum<class "Application.lvclass">)  [unwired: 16 in, 1 out]
          }
        }
      }
      frame "CetoniStop" {
        n196 = call-dynamic "GetCetoniPump.vi"("object in"=w565, "error in (no error)"=w562) -> ("object out"=w566:refnum<class "Application.lvclass">, "CetoniPump"=w561:refnum<class "CetoniPump.lvclass">, "error out"=w559:errorcluster)  [unwired: 15 in]
        n197 = call-dynamic "StopAllPumps.vi"("object in"=w561, "error in (no error)"=w559) -> ("object out"=w560:refnum<class "CetoniPump.lvclass">, "error out"=w558:errorcluster)  [unwired: 16 in]
        n198 = call-dynamic "SetCetoniPump.vi"("object in"=w566, "CetoniPump"=w560, "error in (no error)"=w558) -> ("object out"=w564:refnum<class "Application.lvclass">, "error out"=w563:errorcluster)  [unwired: 15 in]
      }
      frame "CetoniInit" {
        n199 = case shown="True" "Use Cetoni?" {
          tunnel: w571 -> [w573 w584]
          tunnel: [w573 w575] -> w570
          tunnel: [w572 w582] -> w569
          tunnel: w568 -> [w572 w581]
          frame False {
          }
          frame True {
            n200 = call-dynamic "GetCetoniPump.vi"("object in"=w584, "error in (no error)"=w581) -> ("object out"=w585:refnum<class "Application.lvclass">, "CetoniPump"=w580:refnum<class "CetoniPump.lvclass">, "error out"=w578:errorcluster)  [unwired: 15 in]
            n201 = call "CetoniPump_Init.vi"("object in"=w580, "Device Configuration Path"="Device Configuration Path", "error in (no error)"=w578) -> ("object out"=w579:refnum<class "CetoniPump.lvclass">, "error out"=w577:errorcluster)  [unwired: 15 in]
            n202 = call-dynamic "SetCetoniPump.vi"("object in"=w585, "CetoniPump"=w579, "error in (no error)"=w577) -> ("object out"=w583:refnum<class "Application.lvclass">, "error out"=w582:errorcluster)  [unwired: 15 in]
            n203 = call-dynamic "FireStatusEvent.vi"("object in"=w583, "Status"="Cetoni Initialized") -> ("object out"=w575:refnum<class "Application.lvclass">)  [unwired: 16 in, 1 out]
          }
        }
      }
      frame "AdjustPower" {
        # "Do not adjust if wfg is not enabled, only set it for logging purpose"
        n204 = Variant To Data(type=0.0 ("Desired Power"), Variant=w598) -> (data=w596:dbl)  [unwired: 1 in, 1 out]
        n205 = call-dynamic "FireStatusEvent.vi"("object in"=w606, "Status"="Adjusting Power") -> ("object out"=w600:refnum<class "Application.lvclass">)  [unwired: 16 in, 1 out]
        n206 = call-dynamic "GetInstrumentBase.vi"("object in"=w600, "error in (no error)"=w603) -> ("object out"=w595:refnum<class "Application.lvclass">, "InstrumentBase"=w589:refnum<class "InstrumentBase.lvclass">, "error out"=w594:errorcluster)  [unwired: 15 in]
        n207 = call-dynamic "GetWfgEnabled.vi"("object in"=w589) -> ("object out"=w588:refnum<class "InstrumentBase.lvclass">, "WfgEnabled"=w587:cluster{"Ch1":bool, "Ch2":bool})  [unwired: 16 in, 1 out]
        n208 = Unbundle By Name(w587) -> ("Ch1"=w586:bool)
        n209 = case shown="True" w586 {
          tunnel: w596 -> [w607 w619]
          tunnel: w594 -> [w608 w617]
          tunnel: [w611 w616] -> w592
          tunnel: [_ w615] -> w591
          tunnel: [w609 w613] -> w590
          tunnel: w588 -> [w610 w612]
          frame False {
            n210 = call-dynamic "SetDesiredPower(W).vi"("object in"=w610, "DesiredPower(W)"=w607, "error in (no error)"=w608) -> ("object out"=w611:refnum<class "InstrumentBase.lvclass">, "error out"=w609:errorcluster)  [unwired: 15 in]
          }
          frame True {
            n211 = call-dynamic "AdjustPower.vi"("object in"=w612, "DesiredPower(W)"=w619, "error in (no error)"=w617) -> ("object out"=w618:refnum<class "InstrumentBase.lvclass">, "error out"=w614:errorcluster)  [unwired: 15 in]
            n212 = call-dynamic "GetAmplitudeOk.vi"("object in"=w618, "error in (no error)"=w614) -> ("object out"=w616:refnum<class "InstrumentBase.lvclass">, "AmplitudeOk"=w615:bool, "error out"=w613:errorcluster)  [unwired: 15 in]
          }
        }
        "AmplitudeOk" <- w591
        n213 = call-dynamic "SetInstrumentBase.vi"("object in"=w595, "InstrumentBase"=w592, "error in (no error)"=w590) -> ("object out"=w605:refnum<class "Application.lvclass">, "error out"=w604:errorcluster)  [unwired: 15 in]
        n214 = Wait (ms)(milliseconds to wait=u32 200) -> ()  [unwired: 1 out]
        n215 = call-dynamic "FireStatusEvent.vi"("object in"=w605, "Status"="Power Adjusted") -> ("object out"=w602:refnum<class "Application.lvclass">)  [unwired: 16 in, 1 out]
      }
      frame "Wait" {
        n216 = Variant To Data(Variant=w621) -> (data=w620:dbl)  [unwired: 2 in, 1 out]
        n217 = call-dynamic "Wait.vi"("object in"=w625, "Time Target (s)"=w620, "error in (no error)"=w622) -> ("object out"=w624:refnum<class "Application.lvclass">, "error out"=w623:errorcluster)  [unwired: 15 in]
      }
      frame "WfgConfig" {
        n218 = call-dynamic "GetInstrumentBase.vi"("object in"=w637, "error in (no error)"=w628) -> ("object out"=w636:refnum<class "Application.lvclass">, "InstrumentBase"=w633:refnum<class "InstrumentBase.lvclass">, "error out"=w629:errorcluster)  [unwired: 15 in]
        n219 = call-dynamic "ConfigWFG.vi"("object in"=w633, "Config(var)"=w630, "error in (no error)"=w629) -> ("object out"=w632:refnum<class "InstrumentBase.lvclass">, "error out"=w631:errorcluster)  [unwired: 15 in]
        n220 = call-dynamic "SetInstrumentBase.vi"("object in"=w636, "InstrumentBase"=w632, "error in (no error)"=w631) -> ("object out"=w635:refnum<class "Application.lvclass">, "error out"=w634:errorcluster)  [unwired: 15 in]
        n221 = call-dynamic "FireStatusEvent.vi"("object in"=w635, "Status"="WFG Configured") -> ("object out"=w627:refnum<class "Application.lvclass">)  [unwired: 16 in, 1 out]
      }
      frame "WfgChangeFreq" {
        n222 = Variant To Data(error in=w639, type=T14 {"Ch1.Carrier.Frequency (Hz)"=0.0, "Ch2.Carrier.Frequency (Hz)"=0.0} ("Freq Ch1&2"), Variant=w641) -> (data=w638:T14, error out=w640:errorcluster)
        n223 = call-dynamic "GetInstrumentBase.vi"("object in"=w650, "error in (no error)"=w640) -> ("object out"=w649:refnum<class "Application.lvclass">, "InstrumentBase"=w644:refnum<class "InstrumentBase.lvclass">, "error out"=w646:errorcluster)  [unwired: 15 in]
        n224 = call-dynamic "ChangeFreqWFG.vi"("object in"=w644, "Freq Ch1&2"=w638, "error in (no error)"=w646) -> ("object out"=w643:refnum<class "InstrumentBase.lvclass">, "error out"=w645:errorcluster)  [unwired: 15 in]
        n225 = call-dynamic "SetInstrumentBase.vi"("object in"=w649, "InstrumentBase"=w643, "error in (no error)"=w645) -> ("object out"=w648:refnum<class "Application.lvclass">, "error out"=w647:errorcluster)  [unwired: 15 in]
      }
      frame "WfgEnable" {
        n226 = Variant To Data(error in=w653, type=T13 {"Enable Output WFG Ch1"=TRUE, "Enable Output WFG Ch 2"=TRUE} ("OutputEnable 2"), Variant=w655) -> (data=w652:T13, error out=w654:errorcluster)
        n227 = call-dynamic "GetInstrumentBase.vi"("object in"=w663, "error in (no error)"=w654) -> ("object out"=w662:refnum<class "Application.lvclass">, "InstrumentBase"=w659:refnum<class "InstrumentBase.lvclass">, "error out"=w656:errorcluster)  [unwired: 15 in]
        n228 = call-dynamic "EnableWFGOutput.vi"("object in"=w659, "OutputEnable 2"=w652, "error in (no error)"=w656) -> ("object out"=w658:refnum<class "InstrumentBase.lvclass">, "error out"=w657:errorcluster)  [unwired: 15 in]
        n229 = call-dynamic "SetInstrumentBase.vi"("object in"=w662, "InstrumentBase"=w658, "error in (no error)"=w657) -> ("object out"=w661:refnum<class "Application.lvclass">, "error out"=w660:errorcluster)  [unwired: 15 in]
      }
      frame "MSOConfigure" {
        n230 = call-dynamic "GetInstrumentBase.vi"("object in"=w675, "error in (no error)"=w667) -> ("object out"=w674:refnum<class "Application.lvclass">, "InstrumentBase"=w669:refnum<class "InstrumentBase.lvclass">, "error out"=w671:errorcluster)  [unwired: 15 in]
        n231 = call-dynamic "ConfigMSO.vi"("object in"=w669, "variant"=w666, "error in (no error)"=w671) -> ("object out"=w668:refnum<class "InstrumentBase.lvclass">, "error out"=w670:errorcluster)  [unwired: 15 in]
        n232 = call-dynamic "SetInstrumentBase.vi"("object in"=w674, "InstrumentBase"=w668, "error in (no error)"=w670) -> ("object out"=w673:refnum<class "Application.lvclass">, "error out"=w672:errorcluster)  [unwired: 15 in]
        n233 = call-dynamic "FireStatusEvent.vi"("object in"=w673, "Status"="Configuring MSO") -> ("object out"=w665:refnum<class "Application.lvclass">)  [unwired: 16 in, 1 out]
      }
      frame "MSORead" {
        n234 = call-dynamic "GetInstrumentBase.vi"("object in"=w688, "error in (no error)"=w681) -> ("object out"=w687:refnum<class "Application.lvclass">, "InstrumentBase"=w683:refnum<class "InstrumentBase.lvclass">, "error out"=w685:errorcluster)  [unwired: 15 in]
        n235 = call-dynamic "ReadMSO.vi"("object in"=w683, "error in (no error)"=w685) -> ("object out"=w682:refnum<class "InstrumentBase.lvclass">, "Channels array"=w679:waveform(dbl)[], "error out"=w684:errorcluster)  [unwired: 15 in]
        n236 = call-dynamic "SetInstrumentBase.vi"("object in"=w687, "InstrumentBase"=w682, "error in (no error)"=w684) -> ("object out"=w686:refnum<class "Application.lvclass">, "error out"=w677:errorcluster)  [unwired: 15 in]
        n237 = call-dynamic "FireUIEvent.vi"("object in"=w686, "Message"="UpdateMsoData", "Message Data"=w679, "error in (no error)"=w677) -> ("object out"=w680:refnum<class "Application.lvclass">, "error out"=w676:errorcluster)  [unwired: 14 in]
      }
      frame "MSOAutoRange" {
        n238 = call-dynamic "GetInstrumentBase.vi"("object in"=w706, "error in (no error)"=w701) -> ("object out"=w705:refnum<class "Application.lvclass">, "InstrumentBase"=w696:refnum<class "InstrumentBase.lvclass">, "error out"=w695:errorcluster)  [unwired: 15 in]
        n239 = call-dynamic "AutoRangeMSO.vi"("object in"=w696, "error in (no error)"=w695) -> ("object out"=w694:refnum<class "InstrumentBase.lvclass">, "error out"=w692:errorcluster)  [unwired: 16 in]
        n240 = call-dynamic "ReadMSOConfig.vi"("object in"=w694, "error in (no error)"=w692) -> ("object out"=w693:refnum<class "InstrumentBase.lvclass">, "Config"=w690:T18, "error out"=w691:errorcluster)  [unwired: 15 in]
        n241 = call-dynamic "ReadMSO.vi"("object in"=w693, "error in (no error)"=w691) -> ("object out"=w702:refnum<class "InstrumentBase.lvclass">, "Channels array"=w699:waveform(dbl)[], "error out"=w703:errorcluster)  [unwired: 15 in]
        n242 = call-dynamic "SetInstrumentBase.vi"("object in"=w705, "InstrumentBase"=w702, "error in (no error)"=w703) -> ("object out"=w704:refnum<class "Application.lvclass">, "error out"=w697:errorcluster)  [unwired: 15 in]
        n243 = call-dynamic "FireUIEvent.vi"("object in"=w704, "Message"="UpdateMsoData", "Message Data"=w699, "error in (no error)"=w697) -> ("object out"=w700:refnum<class "Application.lvclass">, "error out"=w689:errorcluster)  [unwired: 14 in]
        n244 = local write "Config"(w690) -> ()
      }
      frame "ScanSaveData" {
        n245 = call-dynamic "SaveData.vi"("object in"=w710, "error in (no error)"=w708) -> ("object out"=w709:refnum<class "Application.lvclass">, "error out"=w707:errorcluster)  [unwired: 16 in]
      }
      frame Default {
        # "'Default' case only runs if there is a message that isn't defined in any of the other cases.  Output a programming error."
        n246 = xnode "Error Ring"("parameter 0"=w712) -> ("error out"=w713:errorcluster)
      }
    }
    n247 = call-dynamic "ErrorHandlerMainLoop.vi"("object in"=w18, "error in (no error)"=w21) -> ("object out"=w19:refnum<class "Application.lvclass">, "error out"=w20:errorcluster)  [unwired: 16 in]
  }
  n248 = while {
    tunnel: [w723] -> w9
    shift-right: [w721] -> _
    shift-left: w4 -> [w726]
    tunnel: w13 -> [w725]
    tunnel: w14 -> [w728]
    stop <- w727 stop-if-true
    # "Event Handling Loop"
    n249 = event shown="[6] <UI Event>: User Event" {
      selector: w728 -> [_ _ _ _ _ _ _ _ _ _ _ _ _ _ _ _ _ _ _ _ _ _ _ _ _ _ _ _ _ _ _ _ _ _ _]
      dyn-events: _ -> [_ _ _ _ _ _ _ _ _ _ _ _ _ _ _ _ _ _ _ _ _ _ _ _ _ _ _ _ _ _ _ _ _ _ _]
      timeout: _ -> [_ _ _ _ _ _ _ _ _ _ _ _ _ _ _ _ _ _ _ _ _ _ _ _ _ _ _ _ _ _ _ _ _ _ _]
      tunnel: [_ _ _ _ _ _ _ _ _ _ _ _ _ _ _ _ _ _ _ _ _ _ _ _ _ _ _ _ _ _ _ _ _ _ TRUE ("Discard?")] -> w727
      tunnel: [w731 w740 w741 w743 w750 w755 w762 w860 w868 w876 w889 w894 w900 w905 w910 w915 w920 w925 w930 w936 w941 w946 w952 w957 w965 w969 w973 w977 w981 w985 w990 w995 w1000 w1002 w1007] -> w724
      tunnel: w726 -> [w730 w739 w742 w747 w753 w758 w764 w862 w867 w875 w893 w898 w904 w909 w914 w919 w924 w929 w934 w940 w945 w950 w956 w961 w964 w968 w972 w976 w980 w984 w989 w994 w999 w1006 w1008]
      tunnel: [w729 w738 w742 w746 w752 w757 w763 w861 w867 w875 w892 w897 w903 w908 w913 w918 w923 w928 w933 w939 w944 w949 w955 w960 w963 w967 w971 w975 w979 w983 w988 w993 w998 w1005 w1008] -> w722
      tunnel: w725 -> [w732 w740 w741 w744 w751 w756 w761 w859 w868 w876 w890 w895 w901 w906 w911 w916 w921 w926 w931 w937 w942 w947 w953 w958 w965 w969 w973 w977 w981 w985 w990 w995 w1000 w1001 w1007]
      event Panel Close? {
        # "Send the 'Confirm Quit' message if the user closes the panel of the VI. Discard the event so the 'Confirm Quit' message has a chance to run."
        n250 = event-data() -> ()  [unwired: 1 in, 1 out]
        n251 = call-dynamic "EnqueueMain.vi"("object in"=w730, "Message"="Confirm Quit", "error in (no error)"=w732, "Priority Message? (F)"=TRUE) -> ("object out"=w729:refnum<class "Application.lvclass">, "error out"=w731:errorcluster)  [unwired: 14 in]
        n252 = event-data("Discard?"=TRUE) -> ()  [unwired: 1 in, 1 out]
      }
      event "Freq Ch1&2": Value Change {
        n253 = event-data() -> ()  [unwired: 1 in, 2 out]
        n254 = call-dynamic "EnqueueMain.vi"("object in"=w739, "Message"="WfgChangeFreq", "Message Data"="Freq Ch1&2") -> ("object out"=w738:refnum<class "Application.lvclass">)  [unwired: 15 in, 1 out]
      }
      event Application Instance Close {
        # "#CodeRecommended - When a project closes, all VIs within that project are aborted and leave memory. However, any code placed in this event frame is guaranteed to run to completion, so add any cleanup code that absolutely must happen here."
        n255 = event-data() -> ()  [unwired: 1 in, 1 out]
      }
      event "Configure TEC": Value Change {
        n256 = event-data() -> ()  [unwired: 1 in, 2 out]
        n257 = call-dynamic "EnqueueMain.vi"("object in"=w747, "Message"="MeTecConfigure", "error in (no error)"=w744) -> ("object out"=w746:refnum<class "Application.lvclass">, "error out"=w743:errorcluster)  [unwired: 15 in]
      }
      event "Configure MSO": Value Change {
        n258 = event-data() -> ()  [unwired: 1 in, 2 out]
        n259 = call-dynamic "EnqueueMain.vi"("object in"=w753, "Message"="MSOConfigure", "Message Data"="Config", "error in (no error)"=w751) -> ("object out"=w752:refnum<class "Application.lvclass">, "error out"=w750:errorcluster)  [unwired: 14 in]
      }
      event "AutoRange MSO (Volt)": Value Change {
        n260 = event-data() -> ()  [unwired: 1 in, 2 out]
        n261 = call-dynamic "EnqueueMain.vi"("object in"=w758, "Message"="MSOAutoRange", "error in (no error)"=w756) -> ("object out"=w757:refnum<class "Application.lvclass">, "error out"=w755:errorcluster)  [unwired: 15 in]
      }
      event User Event {
        n262 = event-data() -> ("Message"=w760:string, "Message Data"=w759:variant)  [unwired: 1 in]
        n263 = case shown="\"AutoScaleGraph\"" w760 {
          tunnel: w764 -> [w768 w771 w836 w851 w857]
          tunnel: [w768 w769 w836 w851 w857] -> w763
          tunnel: [w767 w770 w834 w840 w855] -> w762
          tunnel: w761 -> [w766 w773 w833 w839 w854]
          tunnel: w759 -> [_ w772 w835 w841 w856]
          frame "False", Default {
            n264 = Merge Errors(errorcluster {"status"=TRUE, "code"=5005, "source"="INvalid String In Message Handling Loop"} ("error in (no error)"), w766) -> (w767:errorcluster)
          }
          frame "UpdateMsoData" {
            n265 = Variant To Data(error in=w773, type=waveform(dbl)[] [{"t0"=timestamp(0 s since 1904-01-01), "dt"=1e-08, "Y"=array[8192 elements]}, {"t0"=timestamp(0 s since 1904-01-01), "dt"=1e-08, "Y"=array[8192 elements]}] ("Waveform Graph"), Variant=w772) -> (data=w781:waveform(dbl)[], error out=w780:errorcluster)
            "MSO Data WaveForms 2" <- w781
            n266 = for {
              tunnel: [w801] -> w779 mode=concatenating
              shift-right: [w796] -> w777
              shift-left: w780 -> [w797]
              tunnel: [w792] -> w778 mode=concatenating
              tunnel: w781 -> [w791] mode=indexing
              i -> [w807]
              n267 = Increment(x=w807) -> (x+1=w802:i32)
              n268 = call-poly <vilib>:"Extract Single Tone Information.vi"("error in (no error)"=w797, "time signal in"=w791) -> ("error out"=w796:errorcluster, "detected phase (deg)"=w793:dbl, "detected amplitude"=w794:dbl, "detected frequency"=w795:dbl)  [unwired: 4 in, 2 out]
              n269 = Number To Decimal String(number=w802) -> (decimal integer string=w808:string)  [unwired: 1 in]
              n270 = Concatenate Strings("Ch" ("string"), w808) -> (w800:string)
              n271 = Concatenate Strings(w800, "Freq") -> (w804:string)
              n272 = Concatenate Strings(w800, "Amp") -> (w803:string)
              n273 = Concatenate Strings(w800, "Phase") -> (w798:string)
              n274 = Build Array(w795, w794, w793) -> (w792:dbl[])
              n275 = Build Array(w804, w803, w798) -> (w801:string[])
            }
            "Data" <- w779
            "V/Hz/Deg" <- w778
            n276 = Index Array(array=w778) -> (element=w774:dbl)  [unwired: 1 in]
            n277 = case shown="True" "AutoScaleCh1" {
              tunnel: w771 -> [w783 w790]
              tunnel: w777 -> [w784 w787]
              tunnel: [w784 w788] -> w770
              tunnel: "AutoScaleGraph" -> [_ w786]
              tunnel: w774 -> [_ w785]
              tunnel: [w783 w789] -> w769
              frame False {
              }
              frame True {
                n278 = call-dynamic "FireUIEvent.vi"("object in"=w790, "Message"=w786, "Message Data"=w785, "error in (no error)"=w787) -> ("object out"=w789:refnum<class "Application.lvclass">, "error out"=w788:errorcluster)  [unwired: 14 in]
              }
            }
          }
          frame "UpdateTempData" {
            # "prevents the waveform chart from loosing history"
            n279 = Variant To Data(error in=w833, type=waveform(dbl)[] [{"t0"=timestamp(0 s since 1904-01-01), "dt"=1.0, "Y"=[]}] ("appended array"), Variant=w835) -> (data=w822:waveform(dbl)[], error out=w834:errorcluster)
            n280 = property on="Waveform Chart" class="WFChart (strict)"() -> ("History Data"=w825:waveform(dbl)[][])  [unwired: 2 in, 2 out]
            n281 = Index Array(array=w822) -> (element #1=w821:waveform(dbl), element #2=w817:waveform(dbl), element #3=w814:waveform(dbl))  [unwired: 3 in]
            n282 = Index Array(array=w822, index=0) -> (element=w824:waveform(dbl))
            n283 = Unbundle By Name(w821) -> ("t0"=w820:timestamp, "Y"=w819:dbl[])
            n284 = Index Array(array=w825, index (col)=0 ("disabled index (col)")) -> (element=w829:waveform(dbl)[])  [unwired: 1 in]
            n285 = Unbundle By Name(w817) -> ("Y"=w816:dbl[])
            n286 = Unbundle By Name(w814) -> ("Y"=w813:dbl[])
            n287 = Index Array(array=w819) -> (element=w818:dbl)  [unwired: 1 in]
            n288 = Index Array(array=w816) -> (element=w815:dbl)  [unwired: 1 in]
            n289 = Unbundle By Name(w824) -> ("t0"=w823:timestamp)
            n290 = Delete From Array(array=w829) -> (deleted portion=w826:waveform(dbl))  [unwired: 2 in, 1 out]
            n291 = Unbundle By Name(w826) -> ("t0"=w828:timestamp)
            n292 = Index Array(array=w813) -> (element=w812:dbl)  [unwired: 1 in]
            n293 = Greater?(x=w823, y=w828) -> (0:w827:bool)
            n294 = case shown="True" w827 {
              tunnel: w822 -> [_ w837]
              frame False {
              }
              frame True {
                "Waveform Chart" <- w837
              }
            }
            n295 = call "rolling buffer.vi"("mem size"="mem size", "Ch2 2"=w812, "Ch2"=w815, "Ch1"=w818, "current time"=w820) -> ("XY Graph"=→"XY Graph":cluster{timestamp[], dbl[]}[])  [unwired: 6 in]
          }
          frame "AutoScaleGraph" {
            n296 = Variant To Data(error in=w839, type=1.0 ("x"), Variant=w841) -> (data=w846:dbl, error out=w840:errorcluster)
            n297 = Divide(x=1.0, y=w846) -> (x/y=w848:dbl)
            n298 = control-ref of="MSO Data WaveForms 2"() -> (w838:refnum<vi>)
            n299 = Multiply(x=5.0, y=w848) -> (x*y=w844:dbl)
            n300 = property on="Property Node" class="WFGraph (strict)"(reference=w838, "XScale.Maximum"=w844) -> ()  [unwired: 1 in, 2 out]
            n301 = property on="Property Node" class="WFGraph (strict)"(reference=w838, "XScale.ScaleFit"=u8 0 ("X Scale.Scale Fit")) -> ()  [unwired: 1 in, 2 out]
            n302 = property on="Property Node" class="WFGraph (strict)"(reference=w838, "XScale.Minimum"=0.0 ("X Scale.Range:Maximum")) -> ()  [unwired: 1 in, 2 out]
            n303 = property on="Property Node" class="WFGraph (strict)"(reference=w838, "YScale.ScaleFit"=u8 1 ("Y Scale.Scale Fit")) -> ()  [unwired: 1 in, 2 out]
          }
          frame "UpdateStatus" {
            n304 = Variant To Data(error in=w854, type="", Variant=w856) -> (data=→"Status":string, error out=w855:errorcluster)
          }
        }
      }
      event "Start Experiment": Value Change {
        n305 = event-data() -> ()  [unwired: 1 in, 6 out]
        n306 = call-dynamic "EnqueueMain.vi"("object in"=w862, "Message"="StartExperiment", "error in (no error)"=w859) -> ("object out"=w861:refnum<class "Application.lvclass">, "error out"=w860:errorcluster)  [unwired: 15 in]
      }
      event "Fill List": Value Change {
        n307 = event-data() -> ()  [unwired: 1 in, 6 out]
        n308 = for {
          N: "Number of Frequencies" -> [_]
          tunnel: "Freq Start" -> [w870]
          tunnel: "Freq Increment" -> [w872]
          tunnel: [w869] -> w863 mode=indexing
          i -> [w873]
          n309 = Multiply(x=w872, y=w873) -> (x*y=w871:dbl)
          n310 = Add(x=w870, y=w871) -> (x+y=w869:dbl)
        }
        n311 = local write "List of Frequencies (Hz)"(w863) -> ()
      }
      event "Chart Length": Value Change {
        n312 = event-data() -> ()  [unwired: 1 in, 6 out]
        n313 = case shown="\"1 h\"" "Chart Length" {
          frame "60 s", Default {
            n314 = Get Date/Time In Seconds() -> (seconds since 1Jan1904=w880:timestamp)
            n315 = Subtract(x=w880, y=60.0) -> (x-y=w879:timestamp)
            n316 = To Double Precision Float(number=w879) -> (double precision float=w878:dbl)
            n317 = property on="Waveform Chart" class="WFChart (strict)"("XScale.Minimum"=w878) -> ()  [unwired: 2 in, 2 out]
          }
          frame "10 minutes" {
            n318 = Get Date/Time In Seconds() -> (seconds since 1Jan1904=w884:timestamp)
            n319 = Subtract(x=w884, y=600.0) -> (x-y=w882:timestamp)
            n320 = To Double Precision Float(number=w882) -> (double precision float=w881:dbl)
            n321 = property on="Waveform Chart" class="WFChart (strict)"("XScale.Minimum"=w881) -> ()  [unwired: 2 in, 2 out]
          }
          frame "1 h" {
            n322 = Get Date/Time In Seconds() -> (seconds since 1Jan1904=w888:timestamp)
            n323 = Subtract(x=w888, y=3600.0) -> (x-y=w886:timestamp)
            n324 = To Double Precision Float(number=w886) -> (double precision float=w885:dbl)
            n325 = property on="Waveform Chart" class="WFChart (strict)"("XScale.Minimum"=w885) -> ()  [unwired: 2 in, 2 out]
          }
        }
      }
      event "Read MSO": Value Change {
        n326 = event-data() -> ()  [unwired: 1 in, 2 out]
        n327 = call-dynamic "EnqueueMain.vi"("object in"=w893, "Message"="MSORead", "error in (no error)"=w890) -> ("object out"=w892:refnum<class "Application.lvclass">, "error out"=w889:errorcluster)  [unwired: 15 in]
      }
      event "ABORT": Value Change {
        n328 = event-data() -> ()  [unwired: 1 in, 2 out]
        n329 = call-dynamic "EnqueueMain.vi"("object in"=w898, "Message"="Abort", "error in (no error)"=w895) -> ("object out"=w897:refnum<class "Application.lvclass">, "error out"=w894:errorcluster)  [unwired: 15 in]
      }
      event "AdjustPower": Value Change {
        n330 = event-data() -> ()  [unwired: 1 in, 2 out]
        n331 = call-dynamic "EnqueueMain.vi"("object in"=w904, "Message"="AdjustPower", "Message Data"="DesiredPower(W)", "error in (no error)"=w901) -> ("object out"=w903:refnum<class "Application.lvclass">, "error out"=w900:errorcluster)  [unwired: 14 in]
      }
      event "MeasurePower": Value Change {
        n332 = event-data() -> ()  [unwired: 1 in, 2 out]
        n333 = call-dynamic "EnqueueMain.vi"("object in"=w909, "Message"="MeasurePwr", "error in (no error)"=w906) -> ("object out"=w908:refnum<class "Application.lvclass">, "error out"=w905:errorcluster)  [unwired: 15 in]
      }
      event "Refill": Value Change {
        n334 = event-data() -> ()  [unwired: 1 in, 2 out]
        n335 = call-dynamic "EnqueueMain.vi"("object in"=w914, "Message"="CetoniRefill", "error in (no error)"=w911) -> ("object out"=w913:refnum<class "Application.lvclass">, "error out"=w910:errorcluster)  [unwired: 15 in]
      }
      event "ReferenceMove": Value Change {
        n336 = event-data() -> ()  [unwired: 1 in, 2 out]
        n337 = call-dynamic "EnqueueMain.vi"("object in"=w919, "Message"="CetoniRefMove", "error in (no error)"=w916) -> ("object out"=w918:refnum<class "Application.lvclass">, "error out"=w915:errorcluster)  [unwired: 15 in]
      }
      event "Conditional Refill": Value Change {
        n338 = event-data() -> ()  [unwired: 1 in, 2 out]
        n339 = call-dynamic "EnqueueMain.vi"("object in"=w924, "Message"="CetoniCondRefill", "error in (no error)"=w921) -> ("object out"=w923:refnum<class "Application.lvclass">, "error out"=w920:errorcluster)  [unwired: 15 in]
      }
      event "Empty": Value Change {
        n340 = event-data() -> ()  [unwired: 1 in, 2 out]
        n341 = call-dynamic "EnqueueMain.vi"("object in"=w929, "Message"="CetoniEmpty", "error in (no error)"=w926) -> ("object out"=w928:refnum<class "Application.lvclass">, "error out"=w925:errorcluster)  [unwired: 15 in]
      }
      event "Configure Syringe": Value Change {
        n342 = event-data() -> ()  [unwired: 1 in, 2 out]
        n343 = call-dynamic "EnqueueMain.vi"("object in"=w934, "Message"="CetoniConfigure", "error in (no error)"=w931) -> ("object out"=w933:refnum<class "Application.lvclass">, "error out"=w930:errorcluster)  [unwired: 15 in]
      }
      event "ValveControl.Valve Position": Value Change {
        n344 = event-data() -> ()  [unwired: 1 in, 2 out]
        n345 = call-dynamic "EnqueueMain.vi"("object in"=w940, "Message"="CetoniToggleValve", "Message Data"="ValveControl", "error in (no error)"=w937) -> ("object out"=w939:refnum<class "Application.lvclass">, "error out"=w936:errorcluster)  [unwired: 14 in]
      }
      event "Stop pumps": Value Change {
        n346 = event-data() -> ()  [unwired: 1 in, 2 out]
        n347 = call-dynamic "EnqueueMain.vi"("object in"=w945, "Message"="CetoniStop", "error in (no error)"=w942) -> ("object out"=w944:refnum<class "Application.lvclass">, "error out"=w941:errorcluster)  [unwired: 15 in]
      }
      event "Monitor Pump": Value Change {
        n348 = event-data() -> ()  [unwired: 1 in, 2 out]
        n349 = call-dynamic "EnqueueMain.vi"("object in"=w950, "Message"="CetoniMonitor", "error in (no error)"=w947) -> ("object out"=w949:refnum<class "Application.lvclass">, "error out"=w946:errorcluster)  [unwired: 15 in]
      }
      event "Go to Level": Value Change {
        n350 = event-data() -> ()  [unwired: 1 in, 2 out]
        n351 = call-dynamic "EnqueueMain.vi"("object in"=w956, "Message"="CetoniGoToLevel", "Message Data"="GoToLevelSettings", "error in (no error)"=w953) -> ("object out"=w955:refnum<class "Application.lvclass">, "error out"=w952:errorcluster)  [unwired: 14 in]
      }
      event "Run Power Scan": Value Change {
        n352 = event-data() -> ()  [unwired: 1 in, 2 out]
        n353 = call-dynamic "EnqueueMain.vi"("object in"=w961, "Message"="StartPwrScan", "error in (no error)"=w958) -> ("object out"=w960:refnum<class "Application.lvclass">, "error out"=w957:errorcluster)  [unwired: 15 in]
      }
      event "Monitor": Value Change {
        n354 = event-data() -> ()  [unwired: 1 in, 2 out]
        n355 = call-dynamic "EnqueueMain.vi"("object in"=w964, "Message"="MeTecMonitor") -> ("object out"=w963:refnum<class "Application.lvclass">)  [unwired: 16 in, 1 out]
      }
      event "Metec Flush Memory": Value Change {
        n356 = event-data() -> ()  [unwired: 1 in, 2 out]
        n357 = call-dynamic "EnqueueMain.vi"("object in"=w968, "Message"="MeTecFlush") -> ("object out"=w967:refnum<class "Application.lvclass">)  [unwired: 16 in, 1 out]
      }
      event "ResetMtec": Value Change {
        n358 = event-data() -> ()  [unwired: 1 in, 2 out]
        n359 = call-dynamic "EnqueueMain.vi"("object in"=w972, "Message"="MeTecReset") -> ("object out"=w971:refnum<class "Application.lvclass">)  [unwired: 16 in, 1 out]
      }
      event "Initialize System": Value Change {
        n360 = event-data() -> ()  [unwired: 1 in, 2 out]
        n361 = call-dynamic "EnqueueMain.vi"("object in"=w976, "Message"="Initialize") -> ("object out"=w975:refnum<class "Application.lvclass">)  [unwired: 16 in, 1 out]
      }
      event "Image": Value Change {
        n362 = event-data() -> ()  [unwired: 1 in, 2 out]
        n363 = call-dynamic "EnqueueMain.vi"("object in"=w980, "Message"="HamamatsuImage") -> ("object out"=w979:refnum<class "Application.lvclass">)  [unwired: 16 in, 1 out]
      }
      event "Configure": Value Change {
        n364 = event-data() -> ()  [unwired: 1 in, 2 out]
        n365 = call-dynamic "EnqueueMain.vi"("object in"=w984, "Message"="HamamatsuConfigure") -> ("object out"=w983:refnum<class "Application.lvclass">)  [unwired: 16 in, 1 out]
      }
      event "Config WFG": Value Change {
        n366 = event-data() -> ()  [unwired: 1 in, 2 out]
        n367 = call-dynamic "EnqueueMain.vi"("object in"=w989, "Message"="WfgConfig", "Message Data"="Configdatastd") -> ("object out"=w988:refnum<class "Application.lvclass">)  [unwired: 15 in, 1 out]
      }
      event "Configdatastd": Value Change {
        n368 = event-data() -> ()  [unwired: 1 in, 2 out]
        n369 = local read "Configdatastd"() -> (w991:T15)
        n370 = call-dynamic "EnqueueMain.vi"("object in"=w994, "Message"="WfgConfig", "Message Data"=w991) -> ("object out"=w993:refnum<class "Application.lvclass">)  [unwired: 15 in, 1 out]
      }
      event "OutputEnable": Value Change {
        n371 = event-data() -> ()  [unwired: 1 in, 2 out]
        n372 = call-dynamic "EnqueueMain.vi"("object in"=w999, "Message"="WfgEnable", "Message Data"="OutputEnable") -> ("object out"=w998:refnum<class "Application.lvclass">)  [unwired: 15 in, 1 out]
      }
      event "Exit": Value Change {
        n373 = event-data() -> ()  [unwired: 1 in, 1 out]
        n374 = call-dynamic "EnqueueMain.vi"("object in"=w1006, "Message"="Exit", "Message Data"=w1001, "error in (no error)"=w1001, "Priority Message? (F)"=TRUE) -> ("object out"=w1005:refnum<class "Application.lvclass">, "error out"=w1002:errorcluster)  [unwired: 13 in]
      }
      event User Event {
        (unwired) "\"Exit\" button pressed" ("VI Stopped")
        # "The Message Handling Loop processed an \"Exit\" message, which fired this event to stop the Event Handling Loop."
        n375 = event-data() -> ()  [unwired: 1 in, 1 out]
      }
    }
    n376 = call-dynamic "ErrorHandlerEventLoop.vi"("object in"=w722, "error in (no error)"=w724) -> ("object out"=w721:refnum<class "Application.lvclass">, "error out"=w723:errorcluster)  [unwired: 16 in]
  }
  n377 = Merge Errors(w9, w10) -> (w8:errorcluster)
  n378 = call-dynamic "CleanUp.vi"("object in"=w11, "error in (no error)"=w8) -> ("error out"=→"error out":errorcluster)  [unwired: 16 in, 1 out]
